vi "PC_Controller_Launcher.vi"() -> ()   [LabVIEW 2020]
doc: "PC Controller Main VI"
uses:
  TypeDefs/PosZeroOffsets.ctl
  TypeDefs/ReferenceGen.ctl
  RT Target/Controller/TypeDefs/SetRefLocEnum.ctl
  TypeDefs/PosRefOffsets.ctl
  TypeDefs/IncReference.ctl
  TypeDefs/SensorGains.ctl
  TypeDefs/AmplifierGains.ctl
  TypeDefs/CurrSenseZero.ctl
  Components_global/DynamicSignalAnalyzer/TypeDefs/ExcitationSpecs.ctl
  Components_global/DynamicSignalAnalyzer/TypeDefs/CycleSpecs.ctl
  TypeDefs/CurrSenseGains.ctl
  TypeDefs/ControllerGains_UI.ctl
  TypeDefs/ControllerGains_IndAxis.ctl
  TypeDefs/RTdisplayTimedLoop_dt.ctl
  TypeDefs/SensorHposOffset.ctl
  TypeDefs/CoordTransMultipliers.ctl
  Components_global/DynamicSignalAnalyzer/TypeDefs/DSA_TF_params.ctl
  FPGA/Components/FPGA TypeDefs/SelectDirection_Enum.ctl
  TypeDefs/BodeData.ctl
  Components/DisplayWaveform/DisplayWaveforms/DisplayWaveforms.lvclass
  C:/Program Files (x86)/National Instruments/LabVIEW 2020/vi.lib/JKI/JKI SMO/SMO/SMO.lvclass
  C:/Program Files (x86)/National Instruments/LabVIEW 2020/vi.lib/JKI/JKI SMO/SMO.UI/SMO.UI.lvclass
  Components/DisplayWaveform/DisplayWaveforms/Typedefs/Dependencies--Cluster.ctl
  RT Target/Controller/TypeDefs/STMLoopState_enum.ctl
  RT Target/Controller/TypeDefs/FuncGenParams.ctl
  FPGA/Components/FPGA TypeDefs/SelectExcitation_Enum.ctl
  Components_global/DynamicSignalAnalyzer/TypeDefs/DSAconfigCluster.ctl
  Components_global/PlannedMotionSequence/TypeDefs/PlannedMotionSequence.ctl
  Components_global/PlannedMotionSequence/TypeDefs/PlannedMotionSequence_Step.ctl
  Components_global/PlannedMotionSequence/TypeDefs/StepParams.ctl
  Components_global/PlannedMotionSequence/TypeDefs/CtrlEff Params.ctl
  Components_global/PlannedMotionSequence/TypeDefs/PosCtrl Params.ctl
  Components_global/PlannedMotionSequence/TypeDefs/HoldStateParams.ctl
  <vilib>/JKI/JKI SMO/SMO/Typedefs/SMOState --Enum.ctl
  Components_global/Queues/InterProcessQueueCtl.ctl
  TypeDefs/ConfigCluster.ctl
  TypeDefs/GraphInfoCluster.ctl
  Components_global/DynamicSignalAnalyzer/TypeDefs/BodePlot.ctl
  <vilib>/NI/STM/TCP/TCP Read Options.ctl
  <vilib>/NI/STM/TCP/Read Meta Data (TCP Ref).vi
  f38d6d6a-e512-492a-acdc-1d388213210b.vi
  78bd2656-12e6-4809-88cd-6a89556620fb.vi
  5f4b5638-6b16-4865-9ebc-64c862e354be.vi
  83d80429-4559-4d02-b91c-673944bef3a7.vi
  <vilib>/NI/STM/TCP/Get Connection Reference (TCP).vi
  <vilib>/NI/STM/TCP/Read Meta Data (TCP Clst).vi
  <vilib>/JDP Science/JSONtext/JSON text to Variant.vi
  <vilib>/JDP Science/JSONtext/Variant to JSON Text.vi
  <vilib>/NI/STM/TCP/Read Message (TCP).vi
  <vilib>/NI/STM/TCP/Write Message (TCP).vi
  <vilib>/JDP Science/JSONtext/LVClass Serializer/JSONtext LVClass Serializer.lvclass
  <vilib>/NI/STM/NI STM.lvlib
  <vilib>/JKI/JKI SMO/SMO/SMO.lvclass
  <vilib>/JKI/JKI SMO/SMO.UI/SMO.UI.lvclass
  Components_global/Queues/Queues.lvlib
  Components_global/DynamicSignalAnalyzer/DynamicSignalAnalyzer.lvlib
  <vilib>/JDP Science/JSONtext/JSONtext.lvlib
  Components_global/PlannedMotionSequence/PlannedMotionSequence.lvlib
panel:
  in  "Update Chart?":bool
  in  "Clear Chart":bool
  in  "AO Enable?":bool
  in  "Export":bool
  in  "Stop":bool
  out "Status":string
  in  "Tab Control":T1(tab)
  in  "View Raw Pos.":bool
  in  "Update Controller Gains":bool
  in  "Controller Gains":T2={"Z-direction"={"Kp"=1.0, "Ki"=0.0, "fLPF"=0.0}, "ThX-direction"={"Kp"=0.0, "Ki"=0.0, "fLPF"=0.0}, "ThY-direction"={"Kp"=0.0, "Ki"=0.0, "fLPF"=0.0}, "Bow-direction"={"Kp"=0.0, "Ki"=0.0, "fLPF"=0.0}, "B-d - direction"={"Kp"=0.0, "Ki"=0.0, "fLPF"=0.0}}
  in  "Zero Curr. Sense":bool
  in  "Set Pos. Zero":bool
  in  "Update Reference":bool
  in  "Reference Generation":T4
  in  "Run Controller?":bool
  in  "Run Plannned Motion Sequence?":bool
  in  "Sequence JSON File Path":path caption="Path"
  out "Loaded Sequence":string
  out "Bode Data":T8={"Magnitude Bode Plot"={[1.0, 1.2742749857031337, 1.6237767391887217, 2.0691380811147897, 2.636650898730358, 3.3598182862837818, 4.281332398719393, 5.455594781168519, 6.951927961775605, 8.858667904100825, 11.28837891684689, 14.38449888287663, 18.329807108324356, 23.357214690901213, 29.76351441631318, 37.926901907322495, 48.32930238571752, 61.584821106602604, 78.47599703514611, 100.0], [8.190036284839644, 6.422876871403994, 5.062364967545408, 4.022651018777153, 3.220267625701321, 2.6042578837321395, 2.1431756051838486, 1.7956979443459349, 1.5432350752401756, 1.3654027683935595, 1.2417506496398736, 1.1608055133183222, 1.1086862764056675, 1.0725909164599179, 1.0432556265245092, 1.0364066986654934, 1.0216396632894174, 1.0177430021270428, 1.0137984534990414, 1.0067815519527075]}, "Phase Bode Plot"={[1.0, 1.2742749857031337, 1.6237767391887217, 2.0691380811147897, 2.636650898730358, 3.3598182862837818, 4.281332398719393, 5.455594781168519, 6.951927961775605, 8.858667904100825, 11.28837891684689, 14.38449888287663, 18.329807108324356, 23.357214690901213, 29.76351441631318, 37.926901907322495, 48.32930238571752, 61.584821106602604, 78.47599703514611, 100.0], [-81.48463378500874, -79.51768777854348, -77.26541119865844, -74.35073441612305, -70.71358924826187, -66.32524067891468, -60.91360319984072, -54.8342286888728, -48.311197626693605, -41.59636553315517, -34.99300908851906, -29.13860750441638, -24.098834956322154, -19.566458637535703, -14.982365658719985, -13.159615969942717, -9.781179665619796, -8.18372823642157, -6.386288856595014, -4.541305979436174]}}
  in  "Meas. TF params":T9
  in  "Export DSA \ndata?":bool
  in  "Run DSA?":bool
  in  "Cycle Specs":T11={"Cycles To \nSettle (M)"=1, "Cycles To \nCalculate (N)"=2}
  in  "DSA excitation specs":T12={"Initial Freq. [Hz]"=1.0, "Final Freq. [Hz]"=100.0, "# pts. in interval"=20, "Samping Time [us]"=1000.0, "Amplitude"=0.0003, "Offset [V]"=0.0, "Freq Units (F: rad/s, T: Hz)"=TRUE}
  in  "Coord. Trans. Multipliers":T13
  in  "Sensor H-Offset  [mm]":T14={"X"=1.0, "Y"=1.0}
  in  "RT Display Reader Loop Time [us]":T15=1000 caption="Numeric"
  in  "Load\nConfig":bool
  in  "Save\nConfig":bool
  in  "Curr Sense Gain [mA/V]":T16
  in  "Curr Sense Zero [mA]":T17
  in  "Amplifier Gains [V/V]":T18={"G_SE"=1.0, "G_NE"=1.0, "G_NW"=1.0, "G_SW"=1.0, "G_CO"=1.0, "G_CI"=1.0}
  in  "Sensor Gains [um/V]":T19={"G_SE"=1.0, "G_NE"=1.0, "G_NW"=1.0, "G_SW"=1.0, "G_CI"=1.0}
  in  "Pos Zero Offsets [V]":T20
  out "# of display elements \nunpacked (row x col)":i32[](array[numeric]) caption="Numeric"
  out "FPGA Controller Loop Time [us]":dbl caption="Numeric"
  # "Planned Motion Sequence"
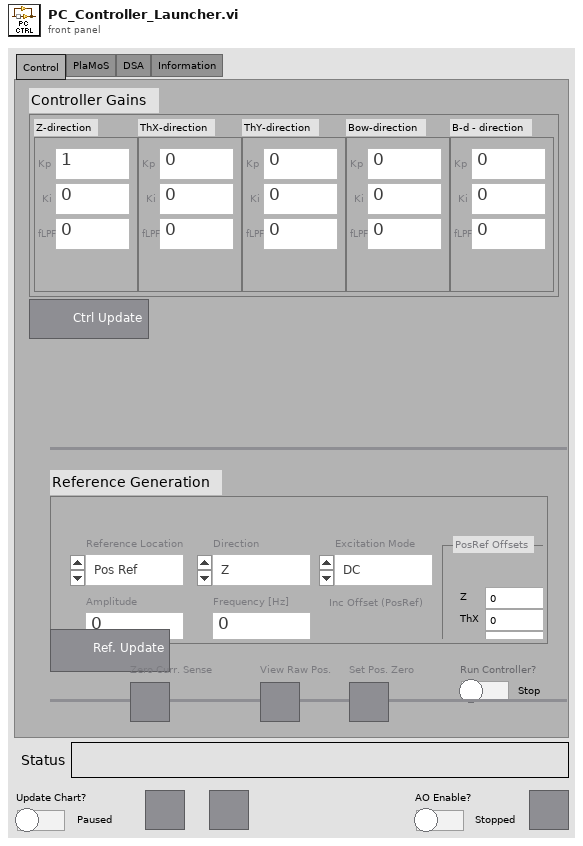
[diagram p1: front panel]
types:
  T1 = enum32{"Control", "PlaMoS", "DSA", "Information"}
  T2 = typedef "ControllerGains_UI.ctl" = cluster{"Z-direction":T3, "ThX-direction":T3, "ThY-direction":T3, "Bow-direction":T3, "B-d - direction":T3}
  T3 = typedef "ControllerGains_IndAxis.ctl" = cluster{"Kp":dbl, "Ki":dbl, "fLPF":dbl}
  T4 = typedef "ReferenceGen.ctl" = cluster{"Reference Location":T5, "Direction":enum16{"Z", "ThX", "ThY", "Bow", "B-d"}, "Excitation Mode":enum16{"DC", "Sine", "Square", "WhiteNoise"}, "Amplitude":dbl, "Frequency [Hz]":dbl, "PosRef Offsets":T6, "Inc Offset (PosRef)":T7}
  T5 = typedef "SetRefLocEnum.ctl" = enum16{"Pos Ref", "Ctrl Eff", "Elec Volt Dist"}
  T6 = typedef "PosRefOffsets.ctl" = cluster{"Z":dbl, "ThX":dbl, "ThY":dbl, "Bow":dbl, "B-d":dbl}
  T7 = typedef "IncReference.ctl" = cluster{"Step":dbl, "Arrow Up":bool, "Arrow Down":bool}
  T8 = typedef "BodeData.ctl" = cluster{"Magnitude Bode Plot":cluster{dbl[], dbl[]}, "Phase Bode Plot":cluster{dbl[], dbl[]}}
  T9 = typedef "DynamicSignalAnalyzer.lvlib/DSA_TF_params.ctl" = cluster{"Direction":T10, "Tras. Func.":enum16{"P", "RR", "C", "*_custom"}}
  T10 = typedef "SelectDirection_Enum.ctl" = enum8{"Z", "ThX", "ThY", "Bow", "B-d"}
  T11 = typedef "DynamicSignalAnalyzer.lvlib/CycleSpecs.ctl" = cluster{"Cycles To \nSettle (M)":i16, "Cycles To \nCalculate (N)":i16}
  T12 = typedef "DynamicSignalAnalyzer.lvlib/ExcitationSpecs.ctl" = cluster{"Initial Freq. [Hz]":dbl, "Final Freq. [Hz]":dbl, "# pts. in interval":i16, "Samping Time [us]":dbl, "Amplitude":dbl, "Offset [V]":dbl, "Freq Units (F: rad/s, T: Hz)":bool}
  T13 = typedef "CoordTransMultipliers.ctl" = cluster{"Z":dbl, "Th":dbl}
  T14 = typedef "SensorHposOffset.ctl" = cluster{"X":dbl, "Y":dbl}
  T15 = typedef "RTdisplayTimedLoop_dt.ctl" = i64
  T16 = typedef "CurrSenseGains.ctl" = cluster{"G_CS":dbl}
  T17 = typedef "CurrSenseZero.ctl" = cluster{"I_SE":dbl, "I_NE":dbl, "I_NW":dbl, "I_SW":dbl, "I_CO":dbl, "I_CI":dbl}
  T18 = typedef "AmplifierGains.ctl" = cluster{"G_SE":dbl, "G_NE":dbl, "G_NW":dbl, "G_SW":dbl, "G_CO":dbl, "G_CI":dbl}
  T19 = typedef "SensorGains.ctl" = cluster{"G_SE":dbl, "G_NE":dbl, "G_NW":dbl, "G_SW":dbl, "G_CI":dbl}
  T20 = typedef "PosZeroOffsets.ctl" = cluster{"V_SE":dbl, "V_NE":dbl, "V_NW":dbl, "V_SW":dbl, "V_CI":dbl}
  T21 = typedef "STMLoopState_enum.ctl" = enum16{"Initialize", "Warm-up", "Run", "ShutDown"}
  T22 = typedef "DisplayWaveform.lvlib/DisplayWaveforms.lvclass/Dependencies--Cluster.ctl" = cluster{"New Value":refnum<user-event>}
  T23 = typedef "SMO.lvclass/Public Events.ctl" = cluster{"Error":refnum<user-event>, "State":refnum<user-event>, "Reserve State":refnum<user-event>}
  T24 = typedef "SMO.UI.lvclass/PublicEvents--Cluster.ctl" = cluster{"UI Hidden":refnum<user-event>, "UI State":refnum<user-event>}
  T25 = typedef "DisplayWaveform.lvlib/DisplayWaveforms.lvclass/PublicEvents--Cluster.ctl" = cluster{"Chart Cleared":refnum<user-event>, "Chart Exported":refnum<user-event>, "ChartParams Set":refnum<user-event>}
  T26 = typedef "NI STM.lvlib/TCP Connection Info.ctl" = cluster{"connection ID":refnum<k5>, "meta data":T27[]}
  T27 = typedef "NI STM.lvlib/MetaDataElement.ctl" = string
  T28 = typedef "Queues.lvlib/Queue Refs.ctl" = cluster{"InterProcessQueue":refnum<queue>}
  T29 = typedef "SMO.lvclass/SMOState --Enum.ctl" = enum16{"unknown", "Created", "Started", "Stopped"}
  T30 = enum32{"Invalid", "Standard", "Closed", "Hidden", "Minimized", "Maximized"}
  T31 = enum32{"invalid app kind", "Development System", "Run Time System", "Student Edition", "Embedded LabVIEW", "Evaluation", "Custom"}
  T32 = typedef "Queues.lvlib/InterProcessQueueCtl.ctl" = cluster{"Command":string, "Data":variant}
  T33 = typedef "FuncGenParams.ctl" = cluster{"Reference Location":T5, "Direction":T10, "Excitation mode":T34, "Amplitude":dbl, "Frequency (periods/tick)":dbl, "PosRef_Offset":dbl[]}
  T34 = typedef "SelectExcitation_Enum.ctl" = enum8{"DC", "Sine", "Square", "WhiteNoise"}
  T35 = enum8{"Enabled", "Disabled", "Disabled and Grayed Out"}
  T36 = typedef "DynamicSignalAnalyzer.lvlib/DSAconfigCluster.ctl" = cluster{"DSA excitation specs":T12, "Cycle Specs":T11, "Meas. TF params":T9}
  T37 = typedef "ConfigCluster.ctl" = cluster{"Controller Gains":T2, "Reference Generation":T4, "RT Display Reader Loop Time [us]":i64, "Sensor Gains [um/V]":T19, "Amplifier Gains [V/V]":T18, "Curr Sense Gain [mA/V]":T16, "Sensor Offset  [mm]":T14, "Coord. Trans. Multipliers":T13, "DSA Config Cluster":T36, "Pos Zero Offsets [V]":T20}
  T38 = enum16{"open", "replace", "create", "open or create", "replace or create", "replace or create with confirmation"}
  T39 = typedef "GraphInfoCluster.ctl" = cluster{"RT Display Reader Loop Time [us]":T15, "Sensor Gains [um/V]":T19, "Sensor H-Offset  [mm]":T14, "Amplifier Gains [V/V]":T18, "Curr Sense Gain [mA/V]":T16}
  T40 = typedef "DynamicSignalAnalyzer.lvlib/BodePlot.ctl" = cluster{"Frequency [Hz]":dbl[], "Magnitude [abs]":dbl[], "Phase [deg]":dbl[]}
  T41 = typedef "PlannedMotionSequence.lvlib/PlannedMotionSequence.ctl" = T42[]
  T42 = typedef "PlannedMotionSequence.lvlib/PlannedMotionSequence_Step.ctl" = cluster{"_Comment":string, "StepParams":T43, "Controller Gains":T2}
  T43 = typedef "PlannedMotionSequence.lvlib/StepParams.ctl" = cluster{"Ctrl State":enum16{"PosCtrl", "CtrlEff", "HoldState"}, "CtrlEff Params":T44, "PosCtrl Params":T45, "HoldState Params":T46}
  T44 = typedef "PlannedMotionSequence.lvlib/CtrlEff Params.ctl" = cluster{"Time [s]":dbl, "U_z":dbl}
  T45 = typedef "PlannedMotionSequence.lvlib/PosCtrl Params.ctl" = cluster{"Velocity [um/s]":dbl, "Starting Z-position [um]":dbl, "Ending Z-position [um]":dbl, "Bow Reference [um]":dbl}
  T46 = typedef "PlannedMotionSequence.lvlib/HoldStateParams.ctl" = cluster{"Time [s]":dbl}
  T47 = cluster{"Core":cluster{"Current VI Reference":refnum<vi>, "Close Panel on Exit?":bool}, "UI switch state":bool, "Export Folder Path":path}
  T48 = cluster{"PosRef Offsets[0]":dbl, "PosRef Offsets[1]":dbl, "PosRef Offsets[2]":dbl, "PosRef Offsets[3]":dbl, "PosRef Offsets[4]":dbl}
  T49 = cluster{"Current VI Reference":refnum<vi>, "Close Panel on Exit?":bool}
  T50 = typedef "ChartParamsCluster.ctl" = cluster{"Chart ScaleMultipliers":cluster{"WF Xscale Multiplier":dbl, "WF Yscale Multiplier":dbl[]}, "Coord Transform Multipliers":cluster{"Z-Multiplier":dbl, "Th-Multiplier":dbl}}
  T51 = typedef "imagedata.ctl" = cluster{"image type":i32, "image depth":i32, "image":u8[], "mask":u8[], "colors":u32[], "Rectangle":cluster{"left":i16, "top":i16, "right":i16, "bottom":i16}}
  T52 = typedef "NI STM.lvlib/TCP Read Options.ctl" = cluster{"ignore timeout error":bool, "timeout ms (1000)":i32}
  T53 = cluster{"V_SE":dbl, "V_NE":dbl, "V_NW":dbl, "V_SW":dbl, "V_CI":dbl}
  T54 = cluster{"I_SE":dbl, "I_NE":dbl, "I_NW":dbl, "I_SW":dbl, "I_CO":dbl, "I_CI":dbl}
  T55 = cluster{"Frequency [Hz]":dbl[], "Magnitude [abs]":dbl[]}
  T56 = cluster{"Frequency [Hz]":dbl[], "Phase [deg]":dbl[]}
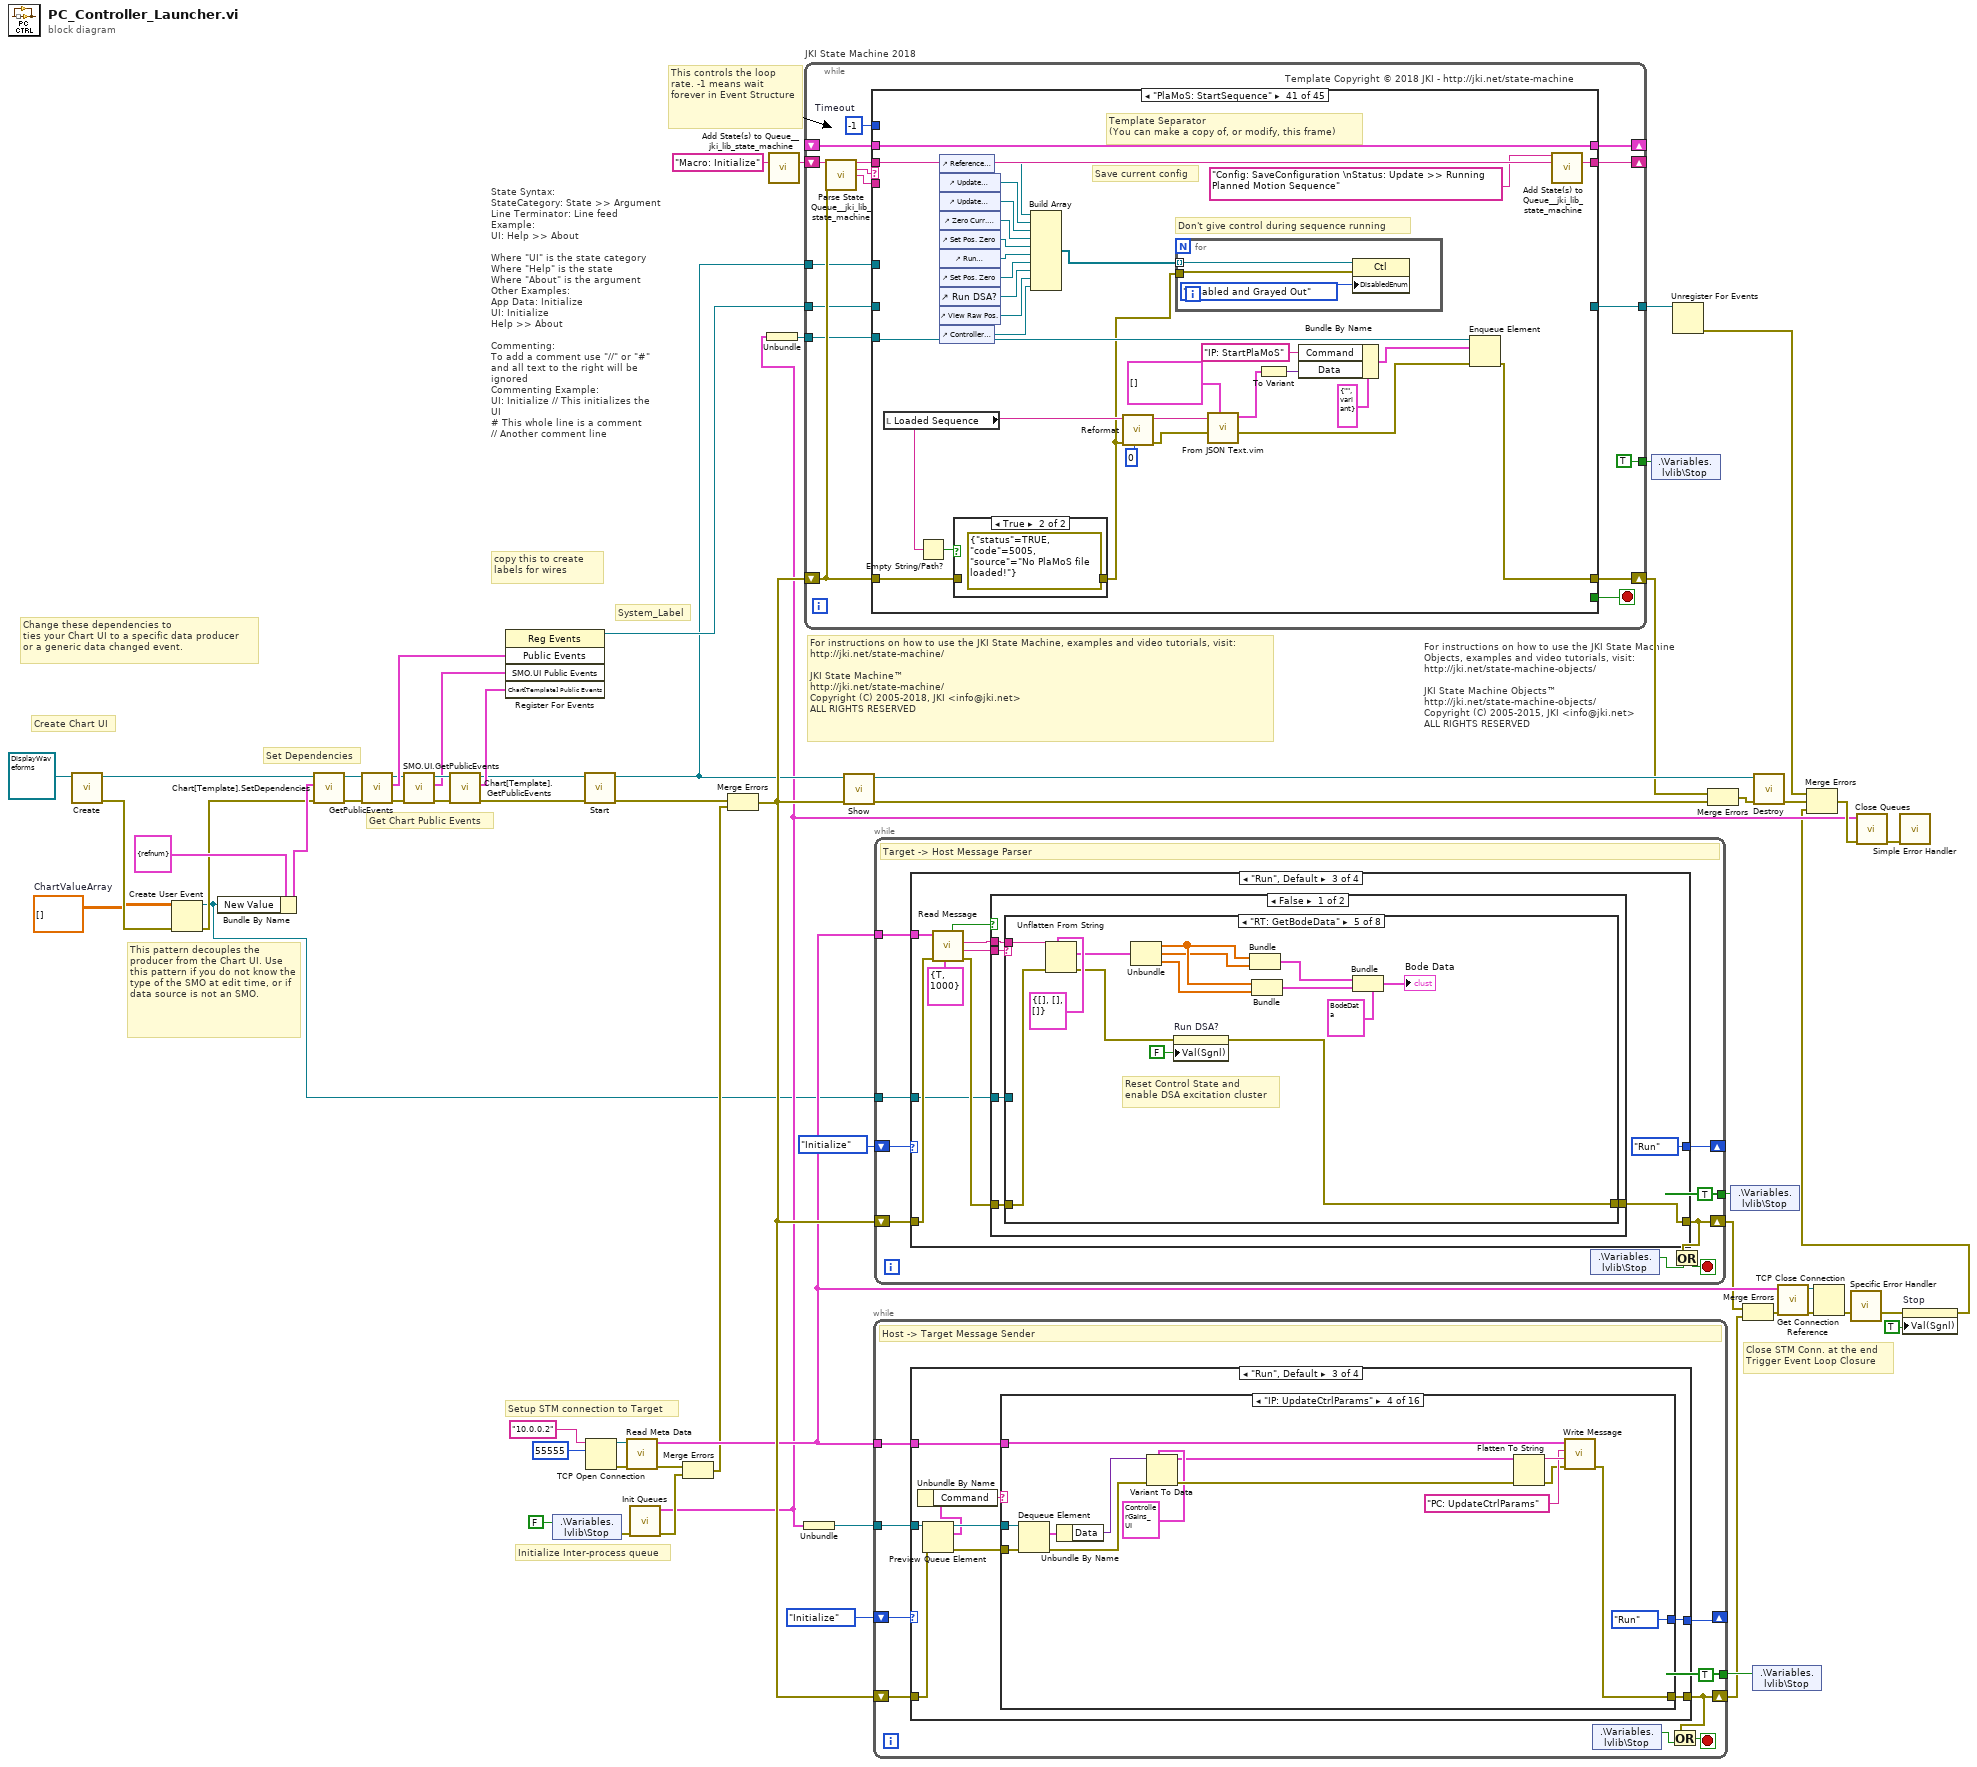
[diagram p0: block diagram]
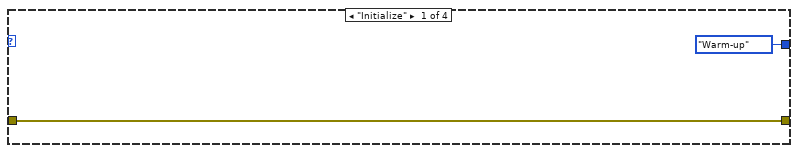
[diagram p2: hidden frame]
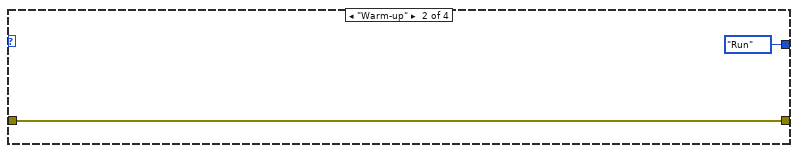
[diagram p3: hidden frame]
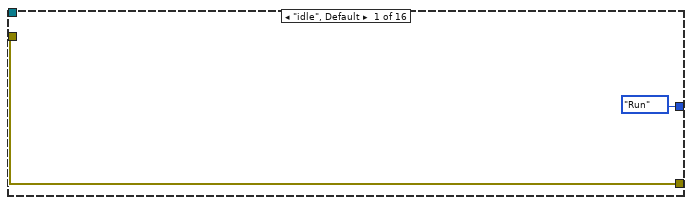
[diagram p4: hidden frame]
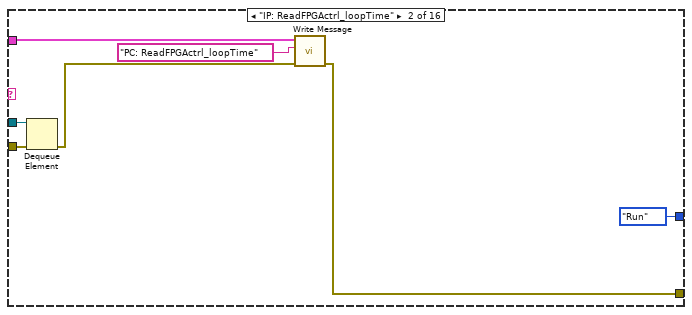
[diagram p5: hidden frame]
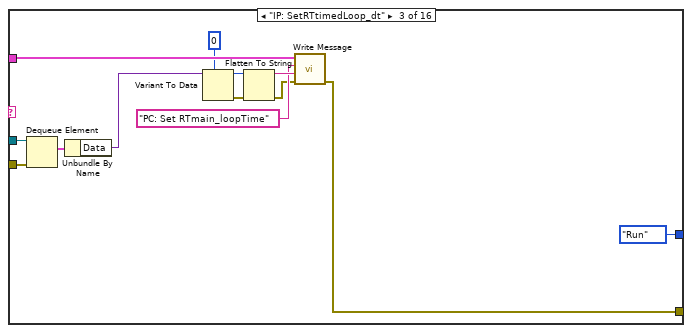
[diagram p6: hidden frame]
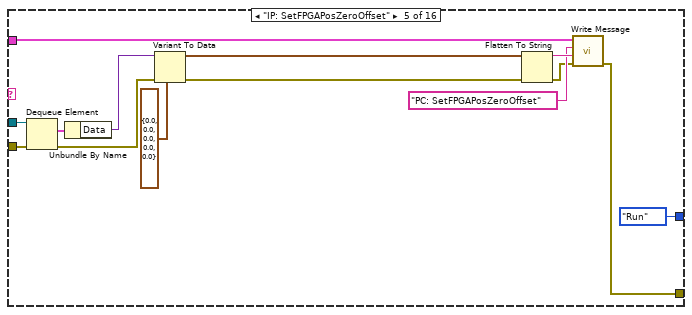
[diagram p7: hidden frame]
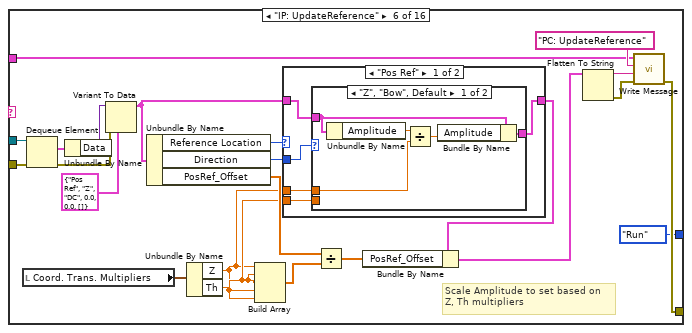
[diagram p8: hidden frame]
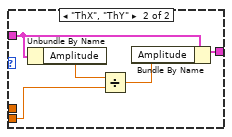
[diagram p9: hidden frame]
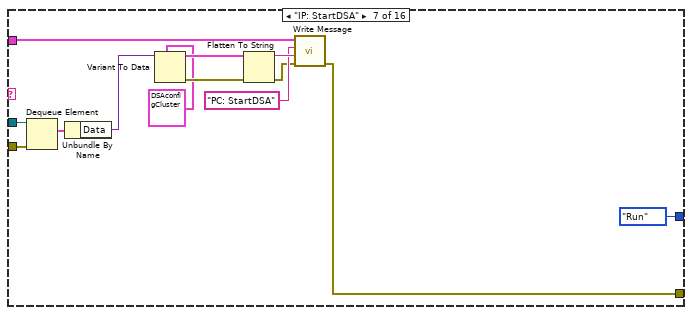
[diagram p11: hidden frame]
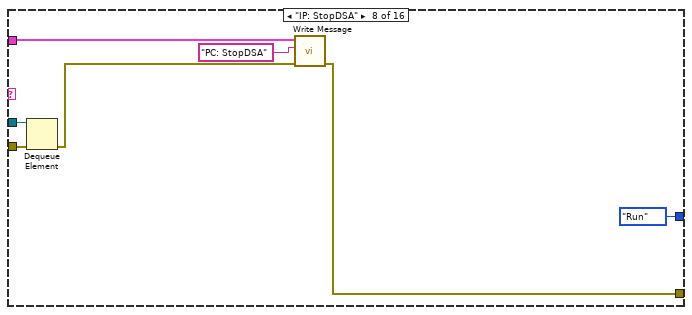
[diagram p12: hidden frame]
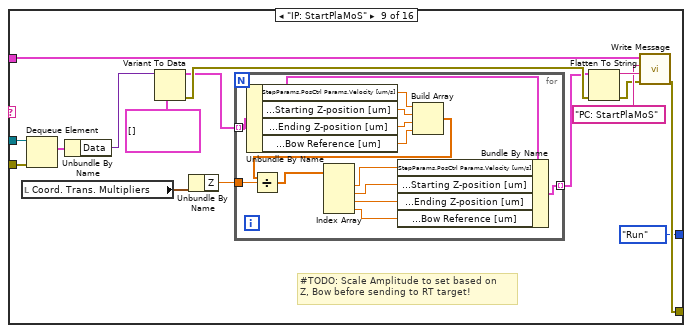
[diagram p13: hidden frame]
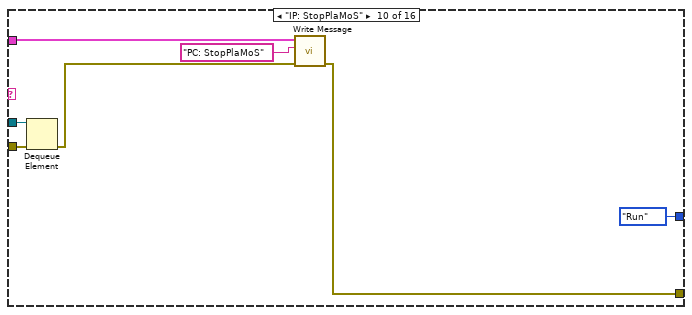
[diagram p14: hidden frame]
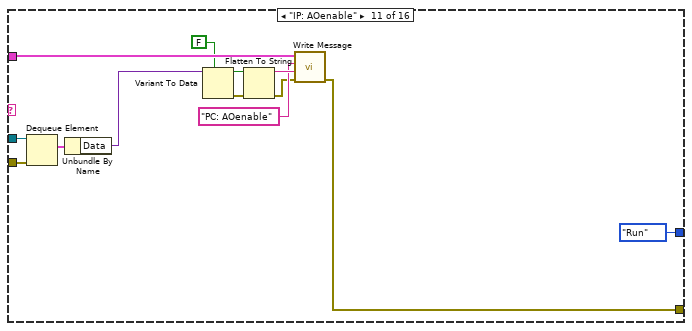
[diagram p15: hidden frame]
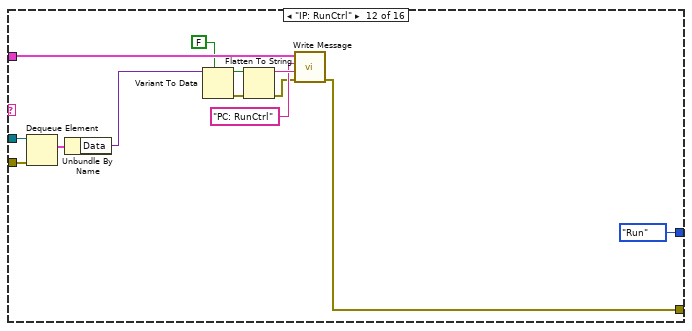
[diagram p16: hidden frame]
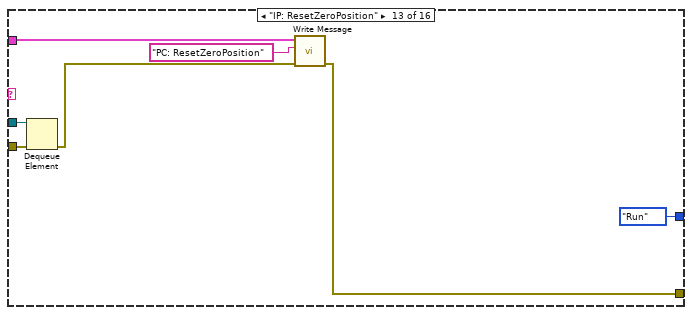
[diagram p17: hidden frame]
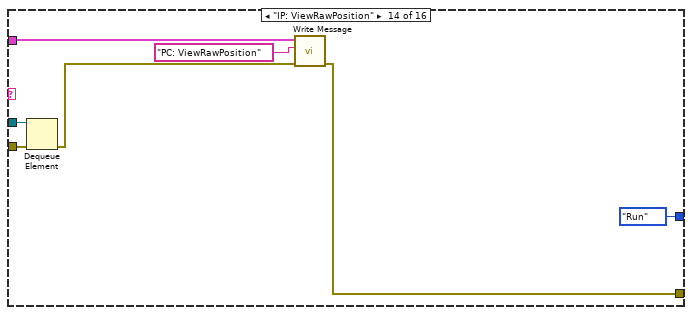
[diagram p18: hidden frame]
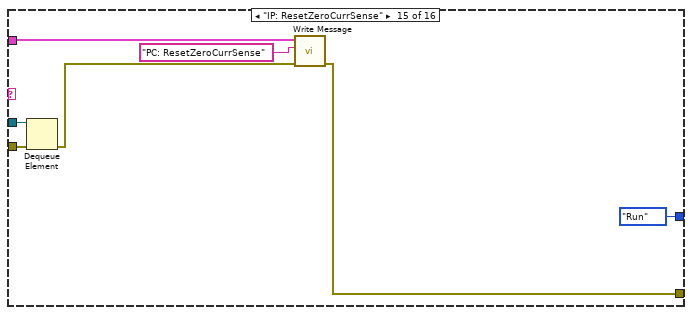
[diagram p19: hidden frame]
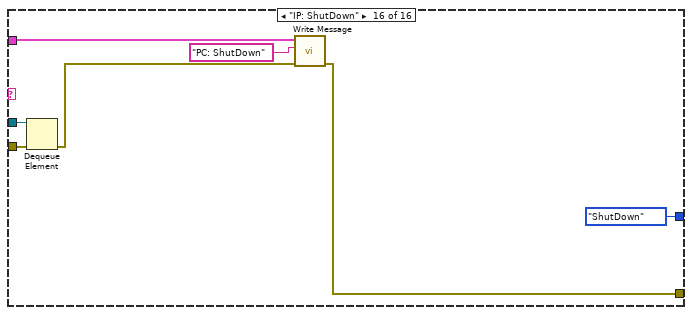
[diagram p20: hidden frame]
diagram:
  w6 = dbl[][] []  # ChartValueArray
  # "Close STM Conn. at the end\nTrigger Event Loop Closure"
  # "Setup STM connection to Target"
  # "Initialize Inter-process queue"
  # "This pattern decouples the producer from the Chart UI. Use this pattern if you do not know the type of the SMO at edit time, or if data source is not an SMO."
  # "For instructions on how to use the JKI State Machine, examples and video tutorials, visit:\nhttp://jki.net/state-machine/\n\nJKI State Machine™\nhttp://jki.net/state-machine/\nCopyright (C) 2005-2018, JKI <info@jki.net>\nALL RIGHTS RESERVED"
  # "State Syntax:\nStateCategory: State >> Argument\nLine Terminator: Line feed\nExample:\nUI: Help >> About\n\nWhere \"UI\" is the state category\nWhere \"Help\" is the state\nWhere \"About\" is the argument\nOther Examples:\nApp Data: Initialize\nUI: Initialize\nHelp >> About\n\nCommenting:\nTo add a comment use \"//\" or \"#\" and all text to the right will be ignored\nCommenting Example:\nUI: Initialize // This initializes the UI\n# This whole line is a comment\n// Another comment line"
  # "copy this to create labels for wires"
  # "This controls the loop rate. -1 means wait forever in Event Structure"
  # "System_Label"
  # "Set Dependencies"
  # "Create Chart UI"
  # "Change these dependencies to\nties your Chart UI to a specific data producer\nor a generic data changed event."
  # "For instructions on how to use the JKI State Machine Objects, examples and video tutorials, visit:\nhttp://jki.net/state-machine-objects/\n\nJKI State Machine Objects™\nhttp://jki.net/state-machine-objects/\nCopyright (C) 2005-2015, JKI <info@jki.net>\nALL RIGHTS RESERVED"
  # "Get Chart Public Events"
  n1 = call <vilib>:"Create.vi"("SMO"=refnum<class "DisplayWaveforms.lvclass"> refnum ("Chart[Template]")) -> ("error out"=w8:errorcluster, "SMO out"=w53:refnum<class "DisplayWaveforms.lvclass">)  [unwired: 8 in, 1 out]
  n2 = Create User Event(user event datatype=w6, error in=w8) -> (user event=w5:refnum<user-event>, error out=w7:errorcluster)
  n3 = Bundle By Name(cluster=T22 {"New Value"=refnum} ("Dependencies"), "New Value"=w5) -> (w51:T22)
  n4 = call "Chart[Template].SetDependencies.vi"("error in (no error)"=w7, "Dependencies"=w51, "DisplayWaveforms"=w53) -> ("error out"=w39:errorcluster, "DisplayWaveforms out"=w50:refnum<class "DisplayWaveforms.lvclass">)  [unwired: 7 in]
  n5 = call <vilib>:"GetPublicEvents.vi"("error in (no error)"=w39, "SMO"=w50) -> ("error out"=w45:errorcluster, "Public Events"=w49:T23, "SMO out"=w47:refnum<class "DisplayWaveforms.lvclass">)  [unwired: 7 in]
  n6 = call <vilib>:"SMO.UI.GetPublicEvents.vi"("error in (no error)"=w45, "SMO.UI"=w47) -> ("error out"=w44:errorcluster, "SMO.UI Public Events"=w43:T24, "SMO.UI out"=w46:refnum<class "DisplayWaveforms.lvclass">)  [unwired: 7 in]
  n7 = call "Chart[Template].GetPublicEvents.vi"("error in (no error)"=w44, "DisplayWaveforms"=w46) -> ("error out"=w40:errorcluster, "Chart[Template] Public Events"=w48:T25, "DisplayWaveforms out"=w41:refnum<class "DisplayWaveforms.lvclass">)  [unwired: 7 in]
  n8 = register-events(w49, w43, w48) -> (reference out=w42:refnum<event-registration>)  [unwired: 2 in, 1 out]
  n9 = shared-variable ".\\Variables.lvlib\\Stop"(FALSE ("Stop")) -> (error out=w30:errorcluster)  [unwired: 1 in]
  n10 = call <vilib>:"Start.vi"("error in (no error)"=w40, "SMO"=w41) -> ("error out"=w25:errorcluster, "SMO out"=w23:refnum<class "DisplayWaveforms.lvclass">)  [unwired: 8 in]
  n11 = TCP Open Connection(address="10.0.0.2" ("Target IP Address"), remote port or service name=u16 55555 ("remote port")) -> (connection ID=w61:refnum<k5>, error out=w60:errorcluster)  [unwired: 1 in, 2 out]
  n12 = call-poly <vilib>:"Read Meta Data.vi"("error in"=w60, "connection ID"=w61) -> ("error out"=w13:errorcluster, "connection info out"=w19:T26)  [unwired: 1 in, 7 out]
  n13 = call "Init Queues.vi"("error in (no error)"=w30) -> ("error out"=w12:errorcluster, "Queue Refs"=w9:T28)  [unwired: 9 in]
  n14 = Merge Errors(w13, w12) -> (w11:errorcluster)
  n15 = Merge Errors(w25, w11) -> (w24:errorcluster)
  n16 = Unbundle(w9) -> ("InterProcessQueue"=w10:refnum<queue>)
  n17 = call <vilib>:"Add State(s) to Queue__jki_lib_state_machine.vi"("State(s) in (\"\")"="Macro: Initialize") -> ("States Out"=w37:string)  [unwired: 14 in]
  n18 = Unbundle(w9) -> ("InterProcessQueue"=w26:refnum<queue>)
  n19 = while "JKI State Machine 2018" {
    shift-right: [w64] -> _
    shift-left: _ -> [w70]
    shift-right: [w72] -> _
    shift-left: w37 -> [w74]
    tunnel: w42 -> [w67]
    tunnel: w23 -> [w66]
    tunnel: [w65] -> w35
    tunnel: [TRUE ("Stop")] -> w33
    shift-right: [w73] -> w4
    shift-left: w24 -> [w68]
    tunnel: w10 -> [w62]
    stop <- w71 stop-if-true
    w69 = -1  # Timeout
    # "Template Copyright © 2018 JKI - http://jki.net/state-machine"
    n20 = call <vilib>:"Parse State Queue__jki_lib_state_machine.vi"("State Queue"=w74, "Error In (no error)"=w68) -> ("Remaining States"=w76:string, "Current State"=w77:string, "Arguments"=w75:string)  [unwired: 11 in]
    n21 = case shown="\"PlaMoS: StartSequence\"" w77 {
      selector: w77 -> [_ _ w279 _ _ _ _ _ _ _ _ _ _ _ _ _ _ _ _ _ _ _ _ _ _ _ _ _ _ _ _ _ _ _ _ _ _ _ _ _ _ _ _ _ _]
      tunnel: w76 -> [w88 w278 w283 w302 w304 w316 w320 w327 w333 w337 w345 w354 w365 w434 w443 w455 w469 w483 w493 w503 w513 w525 w537 w560 w577 w599 w604 w621 w625 w661 w696 w718 w725 w734 w738 w743 w765 w769 w787 w811 w842 w869 w877 w881 w885]
      tunnel: w75 -> [_ _ _ _ _ _ _ _ _ _ _ w349 w359 _ _ _ _ _ _ _ _ _ _ _ _ _ _ _ _ _ w667 _ _ w726 _ _ _ _ _ _ _ _ _ _ _]
      tunnel: w70 -> [w86 w275 w281 w295 w308 w314 w317 _ w328 w334 w343 w352 w361 w431 w437 w453 w460 w471 w491 w501 w511 w523 w535 w558 w571 w596 w601 w619 w622 w659 w666 w721 w722 w731 w735 w740 w762 w766 w785 w809 w840 w867 w874 w878 w882]
      tunnel: [w85 w276 w285 w299 errorcluster {"status"=FALSE, "code"=0, "source"=""} ("error out") w313 w318 w324 w329 w335 w338 w350 w362 w432 w435 w445 w456 w473 w487 w497 w507 w516 w528 w539 w572 w597 w602 w606 w623 w644 w681 w713 w723 w732 w736 w741 w745 w767 w773 w804 w828 w860 w875 w879 w883] -> w73
      tunnel: w68 -> [w84 w276 w284 w299 w307 w313 w318 w324 w330 w335 w340 w351 w363 w432 w436 w446 w457 w474 w486 w496 w506 w517 w529 w540 w573 w597 w602 w608 w623 w654 w682 w714 w723 w732 w736 w741 w761 w767 w775 w804 w824 w861 w875 w879 w883]
      tunnel: [w87 w277 w282 w301 w310 w315 w319 w326 w332 w336 w344 w353 w364 w433 w442 w454 w468 w482 w492 w502 w512 w524 w536 w559 w576 w598 w603 w620 w624 w660 w695 w719 w724 w733 w737 w742 w764 w768 w786 w810 w841 w868 w876 w880 w884] -> w72
      tunnel: [_ _ _ _ _ TRUE _ _ _ _ _ _ _ _ _ _ _ _ _ _ _ _ _ _ _ _ _ _ _ _ _ _ _ _ _ _ _ _ _ _ _ _ _ _ _] -> w71
      tunnel: [w83 w275 w281 w300 w308 w314 w317 w325 w328 w334 w343 w352 w361 w431 w437 w453 w460 w471 w491 w501 w511 w523 w535 w558 w571 w596 w601 w619 w622 w659 w666 w721 w722 w731 w735 w740 w762 w766 w785 w809 w840 w867 w874 w878 w882] -> w64
      tunnel: w69 -> [w82 _ _ _ _ _ _ _ _ _ _ _ _ _ _ _ _ _ _ _ _ _ _ _ _ _ _ _ _ _ _ _ _ _ _ _ _ _ _ _ _ _ _ _ _]
      tunnel: w67 -> [w81 _ _ _ _ w311 _ _ _ _ _ _ _ _ _ _ _ _ _ _ _ _ _ _ _ _ _ _ _ _ _ _ _ _ _ _ _ _ _ _ _ _ _ _ _]
      tunnel: w66 -> [w80 _ _ _ _ _ _ _ _ _ _ _ _ _ _ _ _ _ _ _ _ _ _ _ _ _ _ _ _ _ _ w717 _ _ _ _ _ _ _ _ _ _ _ _ _]
      tunnel: [w79 _ _ _ _ w311 _ _ _ _ _ _ _ _ _ _ _ _ _ _ _ _ _ _ _ _ _ _ _ _ _ _ _ _ _ _ _ _ _ _ _ _ _ _ _] -> w65
      tunnel: w62 -> [w78 _ _ _ _ _ _ _ _ _ _ _ _ _ w438 w447 w461 w475 w485 w495 w505 w518 w530 w542 w574 _ _ w605 _ _ _ _ _ _ _ _ _ _ _ _ w834 w864 _ _ _]
      frame "", "Event Structure", "Idle" {
        # "executes when the state queue is empty"
        n22 = event shown="[16] \"Load Config\": Value Change" {
          selector: w81 -> [_ _ _ _ _ _ _ _ _ _ _ _ _ _ _ _ _ _ _ _ _ _ _]
          dyn-events: [_ _ _ _ _ _ _ _ _ _ _ _ _ _ _ _ _ _ _ _ _ _ _] -> w79
          timeout: w82 -> [_ _ _ _ _ _ _ _ _ _ _ _ _ _ _ _ _ _ _ _ _ _ _]
          tunnel: w88 -> [w92 w98 w105 w109 w114 w119 w124 w129 w147 w165 w173 w179 w194 w204 w211 w215 w220 w228 w237 w249 w259 w263 w270]
          tunnel: [w91 w99 w106 w110 w115 w120 w125 w130 w148 w166 w172 w178 w193 w203 w212 w216 w221 w229 w236 w248 w258 w262 w270] -> w87
          tunnel: w86 -> [w89 w97 w104 w111 w116 w121 w126 w131 w149 w167 w174 w181 w189 w201 w210 w217 w222 w227 w233 w247 w257 w264 w271]
          tunnel: [w90 w93 w101 w107 w112 w117 w123 w128 w146 w164 w175 w182 w196 w202 w207 w213 w218 w224 w230 w239 w250 w265 w272] -> w85
          tunnel: w84 -> [w90 w93 w101 w107 w112 w117 w123 w128 w146 w164 w176 w183 w190 w202 w207 w213 w218 w224 w234 w242 w251 w265 w273]
          tunnel: [w89 w95 w103 w111 w116 w121 w126 w131 w149 w167 w174 w181 w187 w201 w209 w217 w222 w226 w231 w247 w257 w264 w271] -> w83
          tunnel: w80 -> [_ _ _ _ _ _ _ _ _ _ w177 w184 w192 _ _ _ _ _ w235 w243 w252 _ w274]
          tunnel: w78 -> [_ _ _ _ _ _ _ _ _ _ _ _ _ _ _ _ _ _ _ _ _ _ _]
          event Timeout {
            # "README FIRST\nThis VI template should be used by dragging & dropping it from the Functions palette onto the Block Diagram of a new, blank VI, which will place it's contents into the blank VI.\n\nDo not edit the VI found in the palette.  Only edit the state machine after it is placed into your blank VI.\n\nFor instructions on how to use the JKI State Machine, examples and video tutorials, visit:\nhttp://jki.net/state-machine/\n\nDELETE THIS NOTE AFTER READING"
            # "Timeout Frame\n(this will only execute if the Event Structure timeout is >= 0)"
            n23 = event-data() -> ()  [unwired: 1 in, 1 out]
            n24 = call <vilib>:"Add State(s) to Queue__jki_lib_state_machine.vi"("State(s) in (\"\")"=w92) -> ("States Out"=w91:string)  [unwired: 14 in]
          }
          event "AO Enable?": Value Change {
            n25 = event-data() -> ("NewVal"=w96:bool)  [unwired: 1 in, 5 out]
            n26 = Bundle By Name(cluster=w97, "UI switch state"=w96) -> (w95:T47)
            n27 = call <vilib>:"Add State(s) to Queue__jki_lib_state_machine.vi"("State(s) in Front (\"\")"="IP: AOenable" ("State(s) in Front (\"\")"), "State(s) in (\"\")"=w98) -> ("States Out"=w99:string)  [unwired: 13 in]
          }
          event "Run Controller?": Value Change {
            n28 = event-data() -> ("NewVal"=w102:bool)  [unwired: 1 in, 5 out]
            n29 = Bundle By Name(cluster=w104, "UI switch state"=w102) -> (w103:T47)
            n30 = call <vilib>:"Add State(s) to Queue__jki_lib_state_machine.vi"("State(s) in Front (\"\")"="IP: RunController" ("State(s) in Front (\"\")"), "State(s) in (\"\")"=w105) -> ("States Out"=w106:string)  [unwired: 13 in]
          }
          event "Set Pos. Zero": Value Change {
            n31 = event-data() -> ()  [unwired: 1 in, 6 out]
            n32 = call <vilib>:"Add State(s) to Queue__jki_lib_state_machine.vi"("State(s) in Front (\"\")"="IP: ResetZeroPosition", "State(s) in (\"\")"=w109) -> ("States Out"=w110:string)  [unwired: 13 in]
          }
          event "View Raw Pos.": Value Change {
            n33 = event-data() -> ()  [unwired: 1 in, 6 out]
            n34 = call <vilib>:"Add State(s) to Queue__jki_lib_state_machine.vi"("State(s) in Front (\"\")"="IP: ViewRawPosition", "State(s) in (\"\")"=w114) -> ("States Out"=w115:string)  [unwired: 13 in]
          }
          event "Zero Curr. Sense": Value Change {
            n35 = event-data() -> ()  [unwired: 1 in, 6 out]
            n36 = call <vilib>:"Add State(s) to Queue__jki_lib_state_machine.vi"("State(s) in Front (\"\")"="IP: ResetZeroCurrSense", "State(s) in (\"\")"=w119) -> ("States Out"=w120:string)  [unwired: 13 in]
          }
          event "Update Controller Gains": Value Change {
            n37 = event-data() -> ()  [unwired: 1 in, 6 out]
            n38 = call <vilib>:"Add State(s) to Queue__jki_lib_state_machine.vi"("State(s) in Front (\"\")"="IP: UpdateCtrlGains", "State(s) in (\"\")"=w124) -> ("States Out"=w125:string)  [unwired: 13 in]
          }
          event "Update Reference": Value Change {
            n39 = event-data() -> ()  [unwired: 1 in, 6 out]
            n40 = call <vilib>:"Add State(s) to Queue__jki_lib_state_machine.vi"("State(s) in Front (\"\")"="IP: UpdateReference" ("State(s) in Front (\"\")"), "State(s) in (\"\")"=w129) -> ("States Out"=w130:string)  [unwired: 13 in]
          }
          event Value Change {
            n41 = event-data() -> ()  [unwired: 1 in, 6 out]
            n42 = local read "Reference Generation"() -> (w140:T4)
            n43 = Unbundle By Name(w140) -> ("PosRef Offsets"=w144:T6, "Direction"=w142:enum16{"Z", "ThX", "ThY", "Bow", "B-d"}, "Inc Offset (PosRef).Step"=w135:dbl)
            n44 = property on="Reference Generation" class="Clust (strict)"() -> ("Value"=w134:T4)  [unwired: 2 in, 2 out]
            n45 = Bundle By Name(cluster=w134, "Inc Offset (PosRef).Arrow Up"=FALSE ("Inc. Offset.Arrow Down")) -> (w133:T4)
            n46 = Cluster To Array(cluster=w144) -> (array=w143:dbl[])
            n47 = Index Array(array=w143, index=w142) -> (element=w136:dbl)
            n48 = Add(x=w136, y=w135) -> (x+y=w141:dbl)
            n49 = Replace Array Subset(array=w143, new element=w141, index=w142) -> (w139:dbl[])
            n50 = Array To Cluster(array=w139) -> (cluster=w138:T48)
            n51 = Bundle By Name(cluster=w140, "PosRef Offsets"=w138) -> (w137:T4)
            n52 = property on="Reference Generation" class="Clust (strict)"("Value"=w133) -> ()  [unwired: 2 in, 2 out]
            n53 = local write "Reference Generation"(w137) -> ()
            n54 = call <vilib>:"Add State(s) to Queue__jki_lib_state_machine.vi"("State(s) in Front (\"\")"="IP: UpdateReference" ("State(s) in Front (\"\")"), "State(s) in (\"\")"=w147) -> ("States Out"=w148:string)  [unwired: 13 in]
          }
          event Value Change {
            n55 = event-data() -> ()  [unwired: 1 in, 6 out]
            n56 = local read "Reference Generation"() -> (w158:T4)
            n57 = Unbundle By Name(w158) -> ("PosRef Offsets"=w162:T6, "Direction"=w160:enum16{"Z", "ThX", "ThY", "Bow", "B-d"}, "Inc Offset (PosRef).Step"=w153:dbl)
            n58 = property on="Reference Generation" class="Clust (strict)"() -> ("Value"=w152:T4)  [unwired: 2 in, 2 out]
            n59 = Cluster To Array(cluster=w162) -> (array=w161:dbl[])
            n60 = Bundle By Name(cluster=w152, "Inc Offset (PosRef).Arrow Down"=FALSE ("Inc. Offset.Arrow Down")) -> (w151:T4)
            n61 = Index Array(array=w161, index=w160) -> (element=w154:dbl)
            n62 = Subtract(x=w154, y=w153) -> (x-y=w159:dbl)
            n63 = Replace Array Subset(array=w161, new element=w159, index=w160) -> (w157:dbl[])
            n64 = Array To Cluster(array=w157) -> (cluster=w156:T48)
            n65 = Bundle By Name(cluster=w158, "PosRef Offsets"=w156) -> (w155:T4)
            n66 = property on="Reference Generation" class="Clust (strict)"("Value"=w151) -> ()  [unwired: 2 in, 2 out]
            n67 = local write "Reference Generation"(w155) -> ()
            n68 = call <vilib>:"Add State(s) to Queue__jki_lib_state_machine.vi"("State(s) in Front (\"\")"="IP: UpdateReference" ("State(s) in Front (\"\")"), "State(s) in (\"\")"=w165) -> ("States Out"=w166:string)  [unwired: 13 in]
          }
          event "Update Chart?": Value Change {
            n69 = event-data() -> ("NewVal"=w168:bool)  [unwired: 1 in, 5 out]
            n70 = call "UpdateChart.vi"("error in (no error)"=w176, "Update Chart?"=w168, "DisplayWaveforms"=w177) -> ("error out"=w175:errorcluster)  [unwired: 7 in, 1 out]
            n71 = Select(t="Status: Update >> Charts Update Running" ("State(s) in Front (\"\")"), s=w168, f="Status: Update >> Charts Update Paused" ("State(s) in Front (\"\")")) -> (s? t:f=w169:string)
            n72 = call <vilib>:"Add State(s) to Queue__jki_lib_state_machine.vi"("State(s) in Front (\"\")"=w169, "State(s) in (\"\")"=w173) -> ("States Out"=w172:string)  [unwired: 13 in]
          }
          event "Clear Chart": Value Change {
            # "Send Data to UI"
            n73 = event-data() -> ()  [unwired: 1 in, 6 out]
            n74 = call "Clear Chart.vi"("error in (no error)"=w183, "DisplayWaveforms"=w184) -> ("error out"=w182:errorcluster)  [unwired: 8 in, 1 out]
            n75 = call <vilib>:"Add State(s) to Queue__jki_lib_state_machine.vi"("State(s) in Front (\"\")"="Status: Update >> Charts cleared" ("State(s) in Front (\"\")"), "State(s) in (\"\")"=w179) -> ("States Out"=w178:string)  [unwired: 13 in]
          }
          event "Export": Value Change {
            n76 = event-data() -> ()  [unwired: 1 in, 6 out]
            n77 = call "GetExportFolderPath.vi"("error in (no error)"=w190, "DisplayWaveforms"=w192) -> ("error out"=w186:errorcluster, "Export File Folder"=w188:path, "DisplayWaveforms out"=w191:refnum<class "DisplayWaveforms.lvclass">)  [unwired: 7 in]
            n78 = disable-structure shown="Disabled" {
              disable-tunnel: w186 -> [w198 w200]
              disable-tunnel: [w197 w200] -> w185
              frame Disabled {
                # "Also pause chart updates"
                n79 = property on="Update Chart?" class="Bool (strict)"(error in=w198, "Val(Sgnl)"=FALSE ("Value (Signaling)")) -> (error out=w197:errorcluster)  [unwired: 1 in, 1 out]
              }
              frame Enabled {
              }
            }
            n80 = Bundle By Name(cluster=w189, "Export Folder Path"=w188) -> (w187:T47)
            n81 = call "ExportChart.vi"("error in (no error)"=w185, "Export File Folder"=w188, "DisplayWaveforms"=w191) -> ("error out"=w196:errorcluster)  [unwired: 7 in, 1 out]
            n82 = call <vilib>:"Add State(s) to Queue__jki_lib_state_machine.vi"("State(s) in Front (\"\")"="Export: ChartData" ("State(s) in Front (\"\")"), "State(s) in (\"\")"=w194) -> ("States Out"=w193:string)  [unwired: 13 in]
          }
          event "Sequence JSON File Path": Value Change {
            n83 = event-data() -> ()  [unwired: 1 in, 6 out]
            n84 = call <vilib>:"Add State(s) to Queue__jki_lib_state_machine.vi"("State(s) in Front (\"\")"=" PlaMoS: LoadSequence" ("State(s) in Front (\"\")"), "State(s) in (\"\")"=w204) -> ("States Out"=w203:string)  [unwired: 13 in]
          }
          event "Run Plannned Motion Sequence?": Value Change {
            n85 = event-data() -> ("NewVal"=w208:bool)  [unwired: 1 in, 5 out]
            n86 = Bundle By Name(cluster=w210, "UI switch state"=w208) -> (w209:T47)
            n87 = call <vilib>:"Add State(s) to Queue__jki_lib_state_machine.vi"("State(s) in Front (\"\")"="PlaMoS: Start/Stop" ("State(s) in Front (\"\")"), "State(s) in (\"\")"=w211) -> ("States Out"=w212:string)  [unwired: 13 in]
          }
          event "Save\nConfig": Value Change {
            n88 = event-data() -> ()  [unwired: 1 in, 6 out]
            n89 = call <vilib>:"Add State(s) to Queue__jki_lib_state_machine.vi"("State(s) in Front (\"\")"="Config: SaveConfiguration", "State(s) in (\"\")"=w215) -> ("States Out"=w216:string)  [unwired: 13 in]
          }
          event "Load\nConfig": Value Change {
            # "LoadConfiguration file and set zero accordingly"
            n90 = event-data() -> ()  [unwired: 1 in, 6 out]
            n91 = call <vilib>:"Add State(s) to Queue__jki_lib_state_machine.vi"("State(s) in Front (\"\")"="Config: LoadConfiguration\nIP: SetFPGAPosZeroOffset", "State(s) in (\"\")"=w220) -> ("States Out"=w221:string)  [unwired: 13 in]
          }
          event "Run DSA?": Value Change {
            n92 = event-data() -> ("NewVal"=w225:bool)  [unwired: 1 in, 5 out]
            n93 = Bundle By Name(cluster=w227, "UI switch state"=w225) -> (w226:T47)
            n94 = call <vilib>:"Add State(s) to Queue__jki_lib_state_machine.vi"("State(s) in Front (\"\")"="IP: RunDSA" ("State(s) in Front (\"\")"), "State(s) in (\"\")"=w228) -> ("States Out"=w229:string)  [unwired: 13 in]
          }
          event "Export DSA \ndata?": Value Change {
            n95 = event-data() -> ()  [unwired: 1 in, 6 out]
            n96 = call "GetExportFolderPath.vi"("error in (no error)"=w234, "DisplayWaveforms"=w235) -> ("error out"=w230:errorcluster, "Export File Folder"=w232:path)  [unwired: 7 in, 1 out]
            n97 = Bundle By Name(cluster=w233, "Export Folder Path"=w232) -> (w231:T47)
            n98 = call <vilib>:"Add State(s) to Queue__jki_lib_state_machine.vi"("State(s) in Front (\"\")"="Export: DSA Data" ("State(s) in Front (\"\")"), "State(s) in (\"\")"=w237) -> ("States Out"=w236:string)  [unwired: 13 in]
          }
          event "Stop": Value Change {
            # "Stop Communication Process"
            # "Hide UI"
            # "Stop SMO if Stop was pressed"
            # "Exit Button Value Change (pressed) Event\n(this executes Macro: Exit to terminate the VI)"
            n99 = event-data() -> ()  [unwired: 1 in, 6 out]
            n100 = call <vilib>:"Hide.vi"("error in (no error)"=w242, "SMO.UI"=w243) -> ("error out"=w245:errorcluster, "SMO.UI out"=w244:refnum<class "DisplayWaveforms.lvclass">)  [unwired: 8 in]
            n101 = call <vilib>:"Stop.vi"("error in (no error)"=w245, "SMO"=w244) -> ("error out"=w240:errorcluster)  [unwired: 8 in, 1 out]
            n102 = property on="Stop" class="Bool (strict)"(error in=w240, "Value"=FALSE ("Stop")) -> (error out=w239:errorcluster)  [unwired: 1 in, 1 out]
            n103 = call <vilib>:"Add State(s) to Queue__jki_lib_state_machine.vi"("State(s) in Front (\"\")"="Macro: Exit", "State(s) in (\"\")"=w249) -> ("States Out"=w248:string)  [unwired: 13 in]
          }
          event Panel Close? {
            # "Stop SMO if Panel Closed"
            # "Discard the event because we'll close the front panel ourselves in Macro: Exit"
            # "Close Panel button (pressed) Event\n(this executes Macro: Exit to terminate the VI)"
            n104 = event-data() -> ()  [unwired: 1 in, 1 out]
            n105 = call <vilib>:"Hide.vi"("error in (no error)"=w251, "SMO.UI"=w252) -> ("error out"=w253:errorcluster, "SMO.UI out"=w254:refnum<class "DisplayWaveforms.lvclass">)  [unwired: 8 in]
            n106 = call <vilib>:"Stop.vi"("error in (no error)"=w253, "SMO"=w254) -> ("error out"=w250:errorcluster)  [unwired: 8 in, 1 out]
            n107 = event-data("Discard?"=TRUE) -> ()  [unwired: 1 in, 1 out]
            n108 = call <vilib>:"Add State(s) to Queue__jki_lib_state_machine.vi"("State(s) in Front (\"\")"="Macro: Exit", "State(s) in (\"\")"=w259) -> ("States Out"=w258:string)  [unwired: 13 in]
          }
          event User Event {
            n109 = event-data() -> ("SMO State"=w266:T29)  [unwired: 1 in, 4 out]
            n110 = Equal?(x=SMOState_--Enum."Stopped", y=w266) -> (x = y?=w261:bool)
            n111 = case shown="False" w261 {
              tunnel: ["Idle" "Macro: Exit"] -> w260
              frame False {
              }
              frame True {
              }
            }
            n112 = call <vilib>:"Add State(s) to Queue__jki_lib_state_machine.vi"("State(s) in Front (\"\")"=w260, "State(s) in (\"\")"=w263) -> ("States Out"=w262:string)  [unwired: 13 in]
          }
          event User Event {
            # "Stop SMO if UI Closed"
            n113 = event-data() -> ()  [unwired: 1 in, 5 out]
            n114 = call <vilib>:"Stop.vi"("error in (no error)"=w273, "SMO"=w274) -> ("error out"=w272:errorcluster)  [unwired: 8 in, 1 out]
          }
        }
      }
      frame "---------- Core ----------" {
        # "Do not put any code in this frame.\n(it is a separator no-op)"
        n115 = call <vilib>:"Add State(s) to Queue__jki_lib_state_machine.vi"("State(s) in (\"\")"=w278) -> ("States Out"=w277:string)  [unwired: 14 in]
      }
      frame Default {
        w288 = 42 items=["No error", "Argument error", "Memory is full", "Out of zone", "End of file", "File already open", "Generic file I/O error", "File not found", "File permission error", "Disk is full", "Duplicate path", "Too many files open", "System feature not enabled", "Resource file not found", "Cannot add resource", "Resource not found", "Image not found", "Image memory error", "Pen does not exist", "Config type invalid", "Config token not found", "Config parse error", "Config memory error", "Bad external code format", "Bad external code offset", "External code not present", "Null window", "Destroy window error", "Null menu", "Print aborted", "Bad print record", "Print driver error", "Windows error during printing", "Memory error during printing", "Print dialog error", "Generic print error", "Invalid device refnum", "Device not found", "Device parameter error", "Device unit error", "Cannot open device", "Device call aborted", "Generic error", "Cancelled by user", "Object ID too low", "Object ID too high", "Object not in heap", "Unknown heap", "Unknown object (invalid DefProc)", "Unknown object (DefProc not in table)", "Message out of range", "Invalid (null) method", "Unknown message", "Manager call not supported", "Bad address", "Network operation in progress", "Network operation timed out", "Connection is busy", "Network attribute not supported", "Network error", "Address in use", "System out of memory", "Connection aborted", "Connection refused", "Not connected", "Already connected", "Connection closed", "Initialization error (interapplication manager)", "Bad occurrence", "Wait on unbound occurrence handler", "Occurrence queue overflow", "Datalog type conflict", "Unused", "Unrecognized type (interapplication manager)", "Memory corrupt", "Failed to make temporary DLL", "Old CIN version", "Drag socket not found", "Failed to load drop-object", "Failed to register OLE object", "Failed to release OLE object", "Format specifier type mismatch", "Unknown format specifier", "Too few format specifiers", "Too many format specifiers", "Scan failed", "Newer CIN version", "Error converting to variant", "Runtime menu error", "Password tampered", "Variant attribute not found", "Incompatible variant data type", "Event data is not available", "Event Store is not present", "Occurrence is not found", "Event Queue is not created", "Event info is not available", "Refnum passed is NULL", "Error retrieving Class GUID", "Error retrieving CoClass GUID", "Error retrieving TypeLib GUID.", "Bad built application magic bytes.", "Specific driver is different from the specific driver associated with the Logical Name.", "There is no session opened to the class driver.", "Max Error", "MAX - Error with config objects", "MAX - Error loading configuration", "MAX - Group not supported"]
        # "Current State"
        # "Do not delete, rename, or modify this frame.\n(this is used to capture unhandled states and typos)"
        # "Handle mistyped state name (developer tool)"
        n116 = Format Into String(format string="Software Exception: Unhandled State \"%s\"." ("message"), error in=w284, w279) -> (resulting string=w287:string, error out=w286:errorcluster)  [unwired: 1 in]
        n117 = call <vilib>:"Error Cluster From Error Code.vi"("show call chain? (False)"=TRUE, "error in (no error)"=w286, "error message (\"\")"=w287, "error code (0)"=w288) -> ("error out"=w285:errorcluster)  [unwired: 5 in]
        n118 = call <vilib>:"Add State(s) to Queue__jki_lib_state_machine.vi"("State(s) in (\"\")"=w283) -> ("States Out"=w282:string)  [unwired: 14 in]
      }
      frame "Initialize Core Data" {
        # "Do not delete, rename, or modify this frame.\n(this is used to determine panel behavior on exit)"
        # "originally closed?"
        # "exe?"
        # "If panel starts closed or is an EXE, then close it when we exit"
        n119 = property class="VI"() -> ("FP.State"=w292:T30)  [unwired: 2 in, 2 out]
        n120 = property class="App"() -> ("App.Kind"=w298:T31)  [unwired: 2 in, 2 out]
        n121 = control-ref of="Current VI Reference"() -> (w293:refnum<vi>)
        n122 = Equal?(x=w292, y=T30."Closed" ("Front Panel Window:State")) -> (x = y?=w290:bool)
        n123 = Equal?(x=w298, y=T31."Run Time System" ("Application:Kind")) -> (x = y?=w296:bool)
        n124 = Or(x=w290, y=w296) -> (x .or. y?=w294:bool)
        n125 = Bundle By Name(cluster=w295, "Core.Current VI Reference"=w293, "Core.Close Panel on Exit?"=w294) -> (w300:T47)
        n126 = call <vilib>:"Add State(s) to Queue__jki_lib_state_machine.vi"("State(s) in (\"\")"=w302) -> ("States Out"=w301:string)  [unwired: 14 in]
      }
      frame "Error Handler" {
        # "Unhandled Error -- Display it"
        # "Handle any errors here.\nYou can also output any states to clean-up after errors occur"
        # "Clear error"
        n127 = Unbundle By Name(w307) -> ("source"=w305:string)
        n128 = call <vilib>:"General Error Handler.vi"("error in (no error)"=w307) -> ()  [unwired: 10 in, 5 out]
        n129 = Concatenate Strings("/*Post Error States\nStatus: Update >> PC Error: ", w305) -> (w303:string)
        n130 = call <vilib>:"Add State(s) to Queue__jki_lib_state_machine.vi"("State(s) in (\"\")"=w304, "State(s) at Back (\"\")"=w303) -> ("States Out"=w310:string)  [unwired: 13 in]
      }
      frame "Exit" {
        # "Do not put any code in this frame.\n(No errors that occur here will be handled.)"
        n131 = call <vilib>:"Add State(s) to Queue__jki_lib_state_machine.vi"("State(s) in (\"\")"=w316) -> ("States Out"=w315:string)  [unwired: 14 in]
      }
      frame "---------- Data ----------" {
        # "Do not put any code in this frame.\n(It is a separator no-op. You can make a copy of this frame to create a new Data frame)"
        n132 = call <vilib>:"Add State(s) to Queue__jki_lib_state_machine.vi"("State(s) in (\"\")"=w320) -> ("States Out"=w319:string)  [unwired: 14 in]
      }
      frame "Data: Initialize" {
        w321 = path ""  # Export Folder Path
        w322 = T49 {"Current VI Reference"=refnum, "Close Panel on Exit?"=FALSE}  # Core
        w323 = FALSE  # UI switch state
        # "Common Booelan for\nstoring state of any \nUI switch"
        # "Common Booelan for\nstoring state of any \nUI switch"
        # "do not delete - used by framework"
        # "Expand Bundle to add new data elements to shift register data."
        # "Add new data here."
        # "Data names and types of shift register data are defined by this bundle."
        # "Initialize the shift-register data, here.\n(data names are defined by what you wire into the bundle function)"
        n133 = Bundle("Core"=w322, "UI switch state"=w323, "Export Folder Path"=w321) -> (w325:T47)  [unwired: 1 in]
        n134 = call <vilib>:"Add State(s) to Queue__jki_lib_state_machine.vi"("State(s) in (\"\")"=w327) -> ("States Out"=w326:string)  [unwired: 14 in]
      }
      frame "Data: Cleanup" {
        # "Cleanup any data and references, here.\n(this is called automatically, by the Macro: Exit)"
        n135 = Unbundle By Name(w328) -> ("Core.Current VI Reference"=w331:refnum<vi>)
        n136 = Close Reference(reference=w331, error in (no error)=w330) -> (error out=w329:errorcluster)
        n137 = call <vilib>:"Add State(s) to Queue__jki_lib_state_machine.vi"("State(s) in (\"\")"=w333) -> ("States Out"=w332:string)  [unwired: 14 in]
      }
      frame "---------- UI ----------" {
        # "Do not put any code in this frame.\n(It is a separator no-op. You can make a copy of this frame to create a new UI frame)"
        n138 = call <vilib>:"Add State(s) to Queue__jki_lib_state_machine.vi"("State(s) in (\"\")"=w337) -> ("States Out"=w336:string)  [unwired: 14 in]
      }
      frame "UI: Initialize" {
        # "Initialize the User Interface, here.\n(this is called automatically, by the Macro: Init)"
        n139 = disable-structure shown="Enabled" {
          disable-tunnel: w340 -> [w347 _]
          disable-tunnel: [w346 _] -> w339
          frame Enabled {
            # "Reset All front panel controls"
            n140 = control-ref of="This VI"() -> (w348:refnum<vi>)
            n141 = invoke class="VI" method="Default Vals.Reinit All"(reference=w348, error in=w347) -> (error out=w346:errorcluster)  [unwired: 1 in, 2 out]
          }
          frame Disabled {
          }
        }
        n142 = property on="Update Chart?" class="Bool (strict)"(error in=w339, "Val(Sgnl)"=TRUE ("Value (Signaling)")) -> (error out=w338:errorcluster)  [unwired: 1 in, 1 out]
        n143 = call <vilib>:"Add State(s) to Queue__jki_lib_state_machine.vi"("State(s) in Front (\"\")"="Status: Update >> UI Initialized" ("State(s) in Front (\"\")"), "State(s) in (\"\")"=w345) -> ("States Out"=w344:string)  [unwired: 13 in]
      }
      frame "UI: Cursor Set" {
        # "Argument"
        # "Set and Unset Cursor Busy.\n(Usage: \"UI: Cursor Set >> Busy|Idle\")"
        n144 = case shown="\"Idle\", Default" w349 {
          tunnel: w351 -> [w356 w358]
          tunnel: [w355 w357] -> w350
          frame "Idle", Default {
            n145 = call <vilib>:"Unset Busy.vi"("error in (no error)"=w356) -> ("error out"=w355:errorcluster)  [unwired: 10 in]
          }
          frame "Busy" {
            n146 = call <vilib>:"Set Busy.vi"("error in (no error)"=w358) -> ("error out"=w357:errorcluster)  [unwired: 9 in, 1 out]
          }
        }
        n147 = call <vilib>:"Add State(s) to Queue__jki_lib_state_machine.vi"("State(s) in (\"\")"=w354) -> ("States Out"=w353:string)  [unwired: 14 in]
      }
      frame "UI: Front Panel State" {
        # "Argument"
        # "Set Front Panel Open or Closed\n(Usage: \"UI: Front Panel State >> Open|Close\")"
        n148 = Unbundle By Name(w361) -> ("Core.Current VI Reference"=w360:refnum<vi>)
        n149 = case shown="\"Open\", \"Standard\", Default" w359 {
          tunnel: w363 -> [w371 w386 w397 w410 w423]
          tunnel: [w373 w387 w399 w412 w425] -> w362
          tunnel: w360 -> [w372 w384 w398 w411 w424]
          frame "Open", "Standard", Default {
            w366 = T30."Standard" ("State")
            n150 = property class="VI"(reference=w372, error in=w371) -> (reference out=w369:refnum<vi>, error out=w370:errorcluster, "FP.State"=w368:T30)
            n151 = Not Equal?(x=w368, y=w366) -> (x != y?=w367:bool)
            n152 = case shown="False" w367 {
              tunnel: [w377 w379] -> w373
              tunnel: w370 -> [w376 w379]
              tunnel: w369 -> [w375 _]
              tunnel: w366 -> [w374 _]
              frame True {
                n153 = invoke class="VI" method="FP.Open"(reference=w375, error in=w376, "Activate"=TRUE, "State"=w374) -> (error out=w377:errorcluster)  [unwired: 1 in, 4 out]
              }
              frame False {
              }
            }
          }
          frame "Close", "Closed" {
            n154 = property class="VI"(reference=w384, error in=w386) -> (reference out=w383:refnum<vi>, error out=w385:errorcluster, "FP.State"=w381:T30)
            n155 = Not Equal?(x=w381, y=T30."Closed" ("Front Panel Window:State")) -> (x != y?=w380:bool)
            n156 = case shown="True" w380 {
              tunnel: [w388 w391] -> w387
              tunnel: w385 -> [w388 w390]
              tunnel: w383 -> [_ w389]
              frame False {
              }
              frame True {
                n157 = invoke class="VI" method="FP.Close"(reference=w389, error in=w390) -> (error out=w391:errorcluster)  [unwired: 1 in, 2 out]
              }
            }
          }
          frame "Hidden", "Hide" {
            w392 = T30."Hidden" ("State")
            n158 = property class="VI"(reference=w398, error in=w397) -> (reference out=w395:refnum<vi>, error out=w396:errorcluster, "FP.State"=w394:T30)
            n159 = Not Equal?(x=w394, y=w392) -> (x != y?=w393:bool)
            n160 = case shown="True" w393 {
              tunnel: [w403 w404] -> w399
              tunnel: w396 -> [w402 w404]
              tunnel: w395 -> [w401 _]
              tunnel: w392 -> [w400 _]
              frame True {
                n161 = invoke class="VI" method="FP.Open"(reference=w401, error in=w402, "State"=w400) -> (error out=w403:errorcluster)  [unwired: 2 in, 4 out]
              }
              frame False {
              }
            }
          }
          frame "Minimize", "Minimized" {
            w405 = T30."Minimized" ("State")
            n162 = property class="VI"(reference=w411, error in=w410) -> (reference out=w408:refnum<vi>, error out=w409:errorcluster, "FP.State"=w407:T30)
            n163 = Not Equal?(x=w407, y=w405) -> (x != y?=w406:bool)
            n164 = case shown="True" w406 {
              tunnel: [w416 w417] -> w412
              tunnel: w409 -> [w415 w417]
              tunnel: w408 -> [w414 _]
              tunnel: w405 -> [w413 _]
              frame True {
                n165 = invoke class="VI" method="FP.Open"(reference=w414, error in=w415, "State"=w413) -> (error out=w416:errorcluster)  [unwired: 2 in, 4 out]
              }
              frame False {
              }
            }
          }
          frame "Maximize", "Maximized" {
            w418 = T30."Maximized" ("State")
            n166 = property class="VI"(reference=w424, error in=w423) -> (reference out=w421:refnum<vi>, error out=w422:errorcluster, "FP.State"=w420:T30)
            n167 = Not Equal?(x=w420, y=w418) -> (x != y?=w419:bool)
            n168 = case shown="True" w419 {
              tunnel: [w429 w430] -> w425
              tunnel: w422 -> [w428 w430]
              tunnel: w421 -> [w427 _]
              tunnel: w418 -> [w426 _]
              frame True {
                n169 = invoke class="VI" method="FP.Open"(reference=w427, error in=w428, "State"=w426) -> (error out=w429:errorcluster)  [unwired: 2 in, 4 out]
              }
              frame False {
              }
            }
          }
        }
        n170 = call <vilib>:"Add State(s) to Queue__jki_lib_state_machine.vi"("State(s) in (\"\")"=w365) -> ("States Out"=w364:string)  [unwired: 14 in]
      }
      frame "---------- IP ----------" {
        # "Code for inter-process communication \nUse this to send messages via STM to RT target"
        # "Do not put any code in this frame.\n(It is a separator no-op. You can make a copy of this frame to create a new UI frame)"
        n171 = call <vilib>:"Add State(s) to Queue__jki_lib_state_machine.vi"("State(s) in (\"\")"=w434) -> ("States Out"=w433:string)  [unwired: 14 in]
      }
      frame "IP: ReadFPGActrl_loopTime" {
        # "Do not put any code in this frame.\n(It is a separator no-op. You can make a copy of this frame to create a new UI frame)"
        n172 = Bundle By Name(cluster=T32 {"Command"="", "Data"=variant} ("InterProcessQueue"), "Command"="IP: ReadFPGActrl_loopTime") -> (w440:T32)
        n173 = Enqueue Element(queue=w438, element=w440, error in (no error)=w436) -> (error out=w435:errorcluster)  [unwired: 1 in, 2 out]
        n174 = call <vilib>:"Add State(s) to Queue__jki_lib_state_machine.vi"("State(s) in (\"\")"=w443) -> ("States Out"=w442:string)  [unwired: 14 in]
      }
      frame "IP: SetRTtimedLoop_dt" {
        # "During Initialization, Set RT Display Timed Loop Rate"
        # "Do not put any code in this frame.\n(It is a separator no-op. You can make a copy of this frame to create a new UI frame)"
        n175 = local read "RT Display Reader Loop Time [us]"() -> (w444:T15)
        n176 = To Quad Integer(1:w444) -> (0:w448:T15)
        n177 = To Variant(anything=w448) -> (Variant=w449:variant)
        n178 = Bundle By Name(cluster=T32 {"Command"="", "Data"=variant} ("InterProcessQueue"), "Command"="IP: SetRTtimedLoop_dt", "Data"=w449) -> (w451:T32)
        n179 = Enqueue Element(queue=w447, element=w451, error in (no error)=w446) -> (error out=w445:errorcluster)  [unwired: 1 in, 2 out]
        n180 = call <vilib>:"Add State(s) to Queue__jki_lib_state_machine.vi"("State(s) in (\"\")"=w455) -> ("States Out"=w454:string)  [unwired: 14 in]
      }
      frame "IP: AOenable" {
        # "Do not put any code in this frame.\n(It is a separator no-op. You can make a copy of this frame to create a new UI frame)"
        n181 = Unbundle By Name(w460) -> ("UI switch state"=w458:bool)
        n182 = To Variant(anything=w458) -> (Variant=w464:variant)
        n183 = Bundle By Name(cluster=T32 {"Command"="", "Data"=variant} ("InterProcessQueue"), "Command"="IP: AOenable", "Data"=w464) -> (w466:T32)
        n184 = Enqueue Element(queue=w461, element=w466, error in (no error)=w457) -> (error out=w456:errorcluster)  [unwired: 1 in, 2 out]
        n185 = Select(t="Status: Update >> AO enabled" ("State(s) in Front (\"\")"), s=w458, f="Status: Update >> AO disabled" ("State(s) in Front (\"\")")) -> (s? t:f=w459:string)
        n186 = call <vilib>:"Add State(s) to Queue__jki_lib_state_machine.vi"("State(s) in Front (\"\")"=w459, "State(s) in (\"\")"=w469) -> ("States Out"=w468:string)  [unwired: 13 in]
      }
      frame "IP: RunController" {
        # "Do not put any code in this frame.\n(It is a separator no-op. You can make a copy of this frame to create a new UI frame)"
        n187 = Unbundle By Name(w471) -> ("UI switch state"=w470:bool)
        n188 = To Variant(anything=w470) -> (Variant=w481:variant)
        n189 = Bundle By Name(cluster=T32 {"Command"="", "Data"=variant} ("InterProcessQueue"), "Command"="IP: RunCtrl", "Data"=w481) -> (w480:T32)
        n190 = Enqueue Element(queue=w475, element=w480, error in (no error)=w474) -> (error out=w473:errorcluster)  [unwired: 1 in, 2 out]
        n191 = Select(t="Status: Update >> Controller enabled" ("State(s) in Front (\"\")"), s=w470, f="Status: Update >> Controller disabled" ("State(s) in Front (\"\")")) -> (s? t:f=w472:string)
        n192 = call <vilib>:"Add State(s) to Queue__jki_lib_state_machine.vi"("State(s) in Front (\"\")"=w472, "State(s) in (\"\")"=w483) -> ("States Out"=w482:string)  [unwired: 13 in]
      }
      frame "IP: ResetZeroPosition" {
        # "Do not put any code in this frame.\n(It is a separator no-op. You can make a copy of this frame to create a new UI frame)"
        n193 = Bundle By Name(cluster=T32 {"Command"="", "Data"=variant} ("InterProcessQueue"), "Command"="IP: ResetZeroPosition") -> (w489:T32)
        n194 = Enqueue Element(queue=w485, element=w489, error in (no error)=w486) -> (error out=w487:errorcluster)  [unwired: 1 in, 2 out]
        n195 = call <vilib>:"Add State(s) to Queue__jki_lib_state_machine.vi"("State(s) in Front (\"\")"="Status: Update >> Position Zero Offsets updated" ("State(s) in Front (\"\")"), "State(s) in (\"\")"=w493) -> ("States Out"=w492:string)  [unwired: 13 in]
      }
      frame "IP: ViewRawPosition" {
        # "Do not put any code in this frame.\n(It is a separator no-op. You can make a copy of this frame to create a new UI frame)"
        n196 = Bundle By Name(cluster=T32 {"Command"="", "Data"=variant} ("InterProcessQueue"), "Command"="IP: ViewRawPosition") -> (w499:T32)
        n197 = Enqueue Element(queue=w495, element=w499, error in (no error)=w496) -> (error out=w497:errorcluster)  [unwired: 1 in, 2 out]
        n198 = call <vilib>:"Add State(s) to Queue__jki_lib_state_machine.vi"("State(s) in Front (\"\")"="Status: Update >> Position Offsets removed - viewing raw signals" ("State(s) in Front (\"\")"), "State(s) in (\"\")"=w503) -> ("States Out"=w502:string)  [unwired: 13 in]
      }
      frame "IP: ResetZeroCurrSense" {
        # "Do not put any code in this frame.\n(It is a separator no-op. You can make a copy of this frame to create a new UI frame)"
        n199 = Bundle By Name(cluster=T32 {"Command"="", "Data"=variant} ("InterProcessQueue"), "Command"="IP: ResetZeroCurrSense") -> (w509:T32)
        n200 = Enqueue Element(queue=w505, element=w509, error in (no error)=w506) -> (error out=w507:errorcluster)  [unwired: 1 in, 2 out]
        n201 = call <vilib>:"Add State(s) to Queue__jki_lib_state_machine.vi"("State(s) in Front (\"\")"="Status: Update >> Current Sense Zero Offsets updated" ("State(s) in Front (\"\")"), "State(s) in (\"\")"=w513) -> ("States Out"=w512:string)  [unwired: 13 in]
      }
      frame "IP: UpdateCtrlGains" {
        # "Do not put any code in this frame.\n(It is a separator no-op. You can make a copy of this frame to create a new UI frame)"
        n202 = To Variant(anything="Controller Gains") -> (Variant=w519:variant)
        n203 = Bundle By Name(cluster=T32 {"Command"="", "Data"=variant} ("InterProcessQueue"), "Command"="IP: UpdateCtrlParams", "Data"=w519) -> (w521:T32)
        n204 = Enqueue Element(queue=w518, element=w521, error in (no error)=w517) -> (error out=w516:errorcluster)  [unwired: 1 in, 2 out]
        n205 = call <vilib>:"Add State(s) to Queue__jki_lib_state_machine.vi"("State(s) in Front (\"\")"="Status: Update >> Controller Gains Updated" ("State(s) in Front (\"\")"), "State(s) in (\"\")"=w525) -> ("States Out"=w524:string)  [unwired: 13 in]
      }
      frame "IP: SetFPGAPosZeroOffset" {
        # "Do not put any code in this frame.\n(It is a separator no-op. You can make a copy of this frame to create a new UI frame)"
        n206 = To Variant(anything="Pos Zero Offsets [V]") -> (Variant=w531:variant)
        n207 = Bundle By Name(cluster=T32 {"Command"="", "Data"=variant} ("InterProcessQueue"), "Command"="IP: SetFPGAPosZeroOffset", "Data"=w531) -> (w533:T32)
        n208 = Enqueue Element(queue=w530, element=w533, error in (no error)=w529) -> (error out=w528:errorcluster)  [unwired: 1 in, 2 out]
        n209 = call <vilib>:"Add State(s) to Queue__jki_lib_state_machine.vi"("State(s) in Front (\"\")"="Status: Update >> FPGA PosMeas ZeroOffset values set. " ("State(s) in Front (\"\")"), "State(s) in (\"\")"=w537) -> ("States Out"=w536:string)  [unwired: 13 in]
      }
      frame "IP: UpdateReference" {
        # "Convert Frequency from\nHz to periods per tick"
        # "Do not put any code in this frame.\n(It is a separator no-op. You can make a copy of this frame to create a new UI frame)"
        n210 = Unbundle By Name("Reference Generation") -> ("Reference Location"=w551:T5, "Direction"=w550:enum16{"Z", "ThX", "ThY", "Bow", "B-d"}, "Excitation Mode"=w549:enum16{"DC", "Sine", "Square", "WhiteNoise"}, "Amplitude"=w548:dbl, "Frequency [Hz]"=w547:dbl, "PosRef Offsets"=w544:T6)
        n211 = Cluster To Array(cluster=w544) -> (array=w543:dbl[])
        n212 = Multiply(x=w547, y=2.5e-08) -> (x*y=w545:dbl)
        n213 = Bundle By Name(cluster=T33 {"Reference Location"=enum."Pos Ref", "Direction"=enum."Z", "Excitation mode"=enum."DC", "Amplitude"=0.0, "Frequency (periods/tick)"=0.0, "PosRef_Offset"=[]} ("FuncGen Params"), "Reference Location"=w551, "Direction"=w550, "Excitation mode"=w549, "Amplitude"=w548, "Frequency (periods/tick)"=w545, "PosRef_Offset"=w543) -> (w553:T33)
        n214 = To Variant(anything=w553) -> (Variant=w554:variant)
        n215 = Bundle By Name(cluster=T32 {"Command"="", "Data"=variant} ("InterProcessQueue"), "Command"="IP: UpdateReference", "Data"=w554) -> (w556:T32)
        n216 = Enqueue Element(queue=w542, element=w556, error in (no error)=w540) -> (error out=w539:errorcluster)  [unwired: 1 in, 2 out]
        n217 = call <vilib>:"Add State(s) to Queue__jki_lib_state_machine.vi"("State(s) in Front (\"\")"="Status: Update >> Reference Params Updated" ("State(s) in Front (\"\")"), "State(s) in (\"\")"=w560) -> ("States Out"=w559:string)  [unwired: 13 in]
      }
      frame "IP: RunDSA" {
        # "#MAYBE: Split into two cases - StartDSA and Stop DSA\nand call those two cases from this case."
        # "Do not put any code in this frame.\n(It is a separator no-op. You can make a copy of this frame to create a new UI frame)"
        n218 = Unbundle By Name(w571) -> ("UI switch state"=w567:bool)
        n219 = control-ref of="DSA excitation specs"() -> (w563:refnum<vi>)
        n220 = control-ref of="Cycle Specs"() -> (w564:refnum<vi>)
        n221 = Build Array(w563, w564) -> (w562:refnum<vi>[])
        n222 = case shown="False" w567 {
          tunnel: [w580 w592] -> w575
          tunnel: "Cycle Specs" -> [_ w587]
          tunnel: "DSA excitation specs" -> [_ w586]
          tunnel: w562 -> [w578 w585]
          tunnel: "Meas. TF params" -> [_ w584]
          frame False {
            n223 = for {
              tunnel: w578 -> [w583] mode=indexing
              n224 = property class="Clust"(reference=w583, "DisabledEnum"=T35."Enabled" ("Disabled")) -> ()  [unwired: 1 in, 2 out]
            }
            n225 = Bundle By Name(cluster=T32 {"Command"="", "Data"=variant} ("InterProcessQueue"), "Command"="IP: StopDSA") -> (w580:T32)
          }
          frame True {
            n226 = Bundle By Name(cluster=T36 {"DSA excitation specs"={"Initial Freq. [Hz]"=1.0, "Final Freq. [Hz]"=100.0, "# pts. in interval"=20, "Samping Time [us]"=0.0, "Amplitude"=0.0003, "Offset [V]"=0.0, "Freq Units (F: rad/s, T: Hz)"=TRUE}, "Cycle Specs"={"Cycles To \nSettle (M)"=1, "Cycles To \nCalculate (N)"=2}, "Meas. TF params"={"Direction"=enum."Z", "Tras. Func."=enum."P"}} ("DSA Config Cluster"), "DSA excitation specs"=w586, "Cycle Specs"=w587, "Meas. TF params"=w584) -> (w589:T36)
            n227 = for {
              tunnel: w585 -> [w595] mode=indexing
              n228 = property class="Clust"(reference=w595, "DisabledEnum"=T35."Disabled and Grayed Out" ("Disabled")) -> ()  [unwired: 1 in, 2 out]
            }
            n229 = To Variant(anything=w589) -> (Variant=w590:variant)
            n230 = Bundle By Name(cluster=T32 {"Command"="", "Data"=variant} ("InterProcessQueue"), "Command"="IP: StartDSA", "Data"=w590) -> (w592:T32)
          }
        }
        n231 = Select(t="Status: Update >>DSA Running" ("State(s) in Front (\"\")"), s=w567, f="Status: Update >>DSA Stopped" ("State(s) in Front (\"\")")) -> (s? t:f=w569:string)
        n232 = Enqueue Element(queue=w574, element=w575, error in (no error)=w573) -> (error out=w572:errorcluster)  [unwired: 1 in, 2 out]
        n233 = call <vilib>:"Add State(s) to Queue__jki_lib_state_machine.vi"("State(s) in Front (\"\")"=w569, "State(s) in (\"\")"=w577) -> ("States Out"=w576:string)  [unwired: 13 in]
      }
      frame "---------- Macro ----------" {
        # "Do not put any code in this frame.\n(It is a separator no-op. You can make a copy of this frame to create a new Macro frame)"
        n234 = call <vilib>:"Add State(s) to Queue__jki_lib_state_machine.vi"("State(s) in (\"\")"=w599) -> ("States Out"=w598:string)  [unwired: 14 in]
      }
      frame "Macro: Initialize" {
        # "Initialization Macro\n(This is called once, when the VI starts)"
        n235 = call <vilib>:"Add State(s) to Queue__jki_lib_state_machine.vi"("State(s) in Front (\"\")"="Data: Initialize\nInitialize Core Data\n// UI\nUI: Initialize\nUI: Front Panel State >> Open\n// Config\nConfig: LoadConfiguration\nConfig: SendGraphConfig\n// IP\nIP: SetRTtimedLoop_dt \nIP: ReadFPGActrl_loopTime\nIP: SetFPGAPosZeroOffset\nIP: UpdateCtrlGains\nIP: UpdateReference\nIP: RunDSA\n// Status\nStatus: Update >> Controller Initialized", "State(s) in (\"\")"=w604) -> ("States Out"=w603:string)  [unwired: 13 in]
      }
      frame "Macro: Exit" {
        # "Tell RT Target to ShutDown"
        # "Set Stop Global Variable to True"
        # "Exit Macro\n(This is called once, when the VI exits)"
        n236 = Unbundle By Name(w619) -> ("Core.Close Panel on Exit?"=w618:bool)
        n237 = Bundle By Name(cluster=T32 {"Command"="", "Data"=variant} ("InterProcessQueue"), "Command"="IP: ShutDown") -> (w610:T32)
        n238 = Enqueue Element(queue=w605, element=w610, error in (no error)=w608) -> (error out=w607:errorcluster)  [unwired: 1 in, 2 out]
        n239 = shared-variable ".\\Variables.lvlib\\Stop"(TRUE ("Stop"), error in=w607) -> (error out=w606:errorcluster)
        n240 = Select(t="UI: Front Panel State >> Close", s=w618, f="") -> (s? t:f=w615:string)
        n241 = call <vilib>:"Add State(s) to Queue__jki_lib_state_machine.vi"("State(s) in (\"\")"=w615, "State(s) at Back (\"\")"="Data: Cleanup\nPlaMoS: StopSequence\nConfig: SaveConfiguration\nStatus: Update >> Exiting Program\nExit") -> ("States Out"=w613:string)  [unwired: 13 in]
        n242 = call <vilib>:"Add State(s) to Queue__jki_lib_state_machine.vi"("State(s) in Front (\"\")"=w613, "State(s) in (\"\")"=w621) -> ("States Out"=w620:string)  [unwired: 13 in]
      }
      frame "---------- Config ----------" {
        # "Template Separator\n(You can make a copy of, or modify, this frame)"
        n243 = call <vilib>:"Add State(s) to Queue__jki_lib_state_machine.vi"("State(s) in (\"\")"=w625) -> ("States Out"=w624:string)  [unwired: 14 in]
      }
      frame "Config: LoadConfiguration" {
        # "Read \nentire\nfile"
        # "Template Separator\n(You can make a copy of, or modify, this frame)"
        n244 = call <vilib>:"Application Directory.vi"() -> ("Application Directory"=w658:path)
        n245 = Build Path(base path=w658, name or relative path=path "Config.json") -> (appended path=w656:path)
        n246 = Open/Create/Replace File(file path (use dialog)=w656, error in=w654, operation (0:open)=T38."open") -> (refnum out=w651:refnum<file>, error out=w652:errorcluster)  [unwired: 3 in, 1 out]
        n247 = Read from Binary File(8:w652, 10:-1 ("count (1)"), 11:w651) -> (0:w647:errorcluster, 2:w648:string, 3:w650:refnum<file>)  [unwired: 3 in, 1 out]
        n248 = call <vilib>:"Reformat.vi"("Pretty Print Levels"=0, "error in (no error)"=w647, "JSON"=w648) -> ("error out"=w646:errorcluster, "<JSON>"=w649:string)  [unwired: 5 in, 2 out]
        n249 = call "From JSON Text.vim"("Data Type and Default Value"=T37 {"Controller Gains"={"Z-direction"={"Kp"=0.0, "Ki"=0.0, "fLPF"=0.0}, "ThX-direction"={"Kp"=0.0, "Ki"=0.0, "fLPF"=0.0}, "ThY-direction"={"Kp"=0.0, "Ki"=0.0, "fLPF"=0.0}, "Bow-direction"={"Kp"=0.0, "Ki"=0.0, "fLPF"=0.0}, "B-d - direction"={"Kp"=0.0, "Ki"=0.0, "fLPF"=0.0}}, "Reference Generation"={"Reference Location"=enum."Pos Ref", "Direction"=enum."Z", "Excitation Mode"=enum."DC", "Amplitude"=0.0, "Frequency [Hz]"=0.0, "PosRef Offsets"={"Z"=0.0, "ThX"=0.0, "ThY"=0.0, "Bow"=0.0, "B-d"=0.0}, "Inc Offset (PosRef)"={"Step"=0.0, "Arrow Up"=FALSE, "Arrow Down"=FALSE}}, "RT Display Reader Loop Time [us]"=0, "Sensor Gains [um/V]"={"G_SE"=0.0, "G_NE"=0.0, "G_NW"=0.0, "G_SW"=0.0, "G_CI"=0.0}, "Amplifier Gains [V/V]"={"G_SE"=0.0, "G_NE"=0.0, "G_NW"=0.0, "G_SW"=0.0, "G_CO"=0.0, "G_CI"=0.0}, "Curr Sense Gain [mA/V]"={"G_CS"=0.0}, "Sensor Offset  [mm]"={"X"=1.0, "Y"=1.0}, "Coord. Trans. Multipliers"={"Z"=0.0, "Th"=0.0}, "DSA Config Cluster"={"DSA excitation specs"={"Initial Freq. [Hz]"=0.0, "Final Freq. [Hz]"=0.0, "# pts. in interval"=0, "Samping Time [us]"=0.0, "Amplitude"=0.0, "Offset [V]"=0.0, "Freq Units (F: rad/s, T: Hz)"=FALSE}, "Cycle Specs"={"Cycles To \nSettle (M)"=0, "Cycles To \nCalculate (N)"=0}, "Meas. TF params"={"Direction"=enum."Z", "Tras. Func."=enum."P"}}, "Pos Zero Offsets [V]"={"V_SE"=0.0, "V_NE"=0.0, "V_NW"=0.0, "V_SW"=0.0, "V_CI"=0.0}} ("Config Cluster"), "error in (no error)"=w646, "JSON"=w649) -> ("error out"=w633:errorcluster, "Data out"=w641:T37)  [unwired: 7 in]
        n250 = Unbundle By Name(w641) -> ("Controller Gains"=w629:T2, "Reference Generation"=w638:T4, "RT Display Reader Loop Time [us]"=w639:i64, "Sensor Gains [um/V]"=w637:T19, "Amplifier Gains [V/V]"=w636:T18, "Curr Sense Gain [mA/V]"=w635:T16, "Sensor Offset  [mm]"=w632:T14, "Coord. Trans. Multipliers"=w630:T13, "DSA Config Cluster"=w631:T36, "Pos Zero Offsets [V]"=w628:T20)
        n251 = Close File(refnum=w650, error in=w647) -> (error out=w645:errorcluster)  [unwired: 1 out]
        n252 = Merge Errors(w633, w645) -> (w644:errorcluster)
        n253 = Unbundle(w631) -> ("DSA excitation specs"=w634:T12, "Cycle Specs"=w627:T11, "Meas. TF params"=w626:T9)
        n254 = local write "Controller Gains"(w629) -> ()
        n255 = local write "Reference Generation"(w638) -> ()
        n256 = local write "RT Display Reader Loop Time [us]"(w639) -> ()
        n257 = local write "Sensor Gains [um/V]"(w637) -> ()
        n258 = local write "Amplifier Gains [V/V]"(w636) -> ()
        n259 = local write "Curr Sense Gain [mA/V]"(w635) -> ()
        n260 = local write "Sensor H-Offset  [mm]"(w632) -> ()
        n261 = local write "Coord. Trans. Multipliers"(w630) -> ()
        n262 = local write "DSA excitation specs"(w634) -> ()
        n263 = local write "Cycle Specs"(w627) -> ()
        n264 = local write "Meas. TF params"(w626) -> ()
        n265 = local write "Pos Zero Offsets [V]"(w628) -> ()
        n266 = call <vilib>:"Add State(s) to Queue__jki_lib_state_machine.vi"("State(s) in Front (\"\")"="\nStatus: Update >> Params loaded from Config file" ("State(s) in Front (\"\")"), "State(s) in (\"\")"=w661) -> ("States Out"=w660:string)  [unwired: 13 in]
      }
      frame "Config: SaveConfiguration" {
        # "Template Separator\n(You can make a copy of, or modify, this frame)"
        n267 = case shown="\"idle\", Default" w667 {
          tunnel: [w697 w701] -> w694
          tunnel: w666 -> [w700 _]
          frame "Export" {
            # "Use export folder path."
            n268 = Unbundle By Name(w700) -> ("Export Folder Path"=w699:path)
            n269 = Build Path(base path=w699, name or relative path=path "Config.json") -> (appended path=w697:path)
          }
          frame "idle", Default {
            # "Use Config file in project folder"
            n270 = call <vilib>:"Application Directory.vi"() -> ("Application Directory"=w703:path)
            n271 = Build Path(base path=w703, name or relative path=path "Config.json") -> (appended path=w701:path)
          }
        }
        n272 = local read "Controller Gains"() -> (w665:T2)
        n273 = local read "Reference Generation"() -> (w679:T4)
        n274 = local read "RT Display Reader Loop Time [us]"() -> (w678:T15)
        n275 = local read "Sensor Gains [um/V]"() -> (w677:T19)
        n276 = local read "Amplifier Gains [V/V]"() -> (w676:T18)
        n277 = local read "Curr Sense Gain [mA/V]"() -> (w675:T16)
        n278 = local read "Sensor H-Offset  [mm]"() -> (w670:T14)
        n279 = local read "Coord. Trans. Multipliers"() -> (w668:T13)
        n280 = local read "DSA excitation specs"() -> (w674:T12)
        n281 = local read "Cycle Specs"() -> (w673:T11)
        n282 = local read "Meas. TF params"() -> (w664:T9)
        n283 = local read "Pos Zero Offsets [V]"() -> (w663:T20)
        n284 = Bundle(cluster=T36 {"DSA excitation specs"={"Initial Freq. [Hz]"=1.0, "Final Freq. [Hz]"=100.0, "# pts. in interval"=20, "Samping Time [us]"=0.0, "Amplitude"=0.0003, "Offset [V]"=0.0, "Freq Units (F: rad/s, T: Hz)"=TRUE}, "Cycle Specs"={"Cycles To \nSettle (M)"=1, "Cycles To \nCalculate (N)"=2}, "Meas. TF params"={"Direction"=enum."Z", "Tras. Func."=enum."P"}} ("DSA Config Cluster"), "DSA excitation specs"=w674, "Cycle Specs"=w673, "Meas. TF params"=w664) -> (w669:T36)
        n285 = Open/Create/Replace File(file path (use dialog)=w694, error in=w682, operation (0:open)=T38."open or create") -> (refnum out=w687:refnum<file>, error out=w662:errorcluster)  [unwired: 3 in, 1 out]
        n286 = Bundle(cluster=T37 {"Controller Gains"={"Z-direction"={"Kp"=0.0, "Ki"=0.0, "fLPF"=0.0}, "ThX-direction"={"Kp"=0.0, "Ki"=0.0, "fLPF"=0.0}, "ThY-direction"={"Kp"=0.0, "Ki"=0.0, "fLPF"=0.0}, "Bow-direction"={"Kp"=0.0, "Ki"=0.0, "fLPF"=0.0}, "B-d - direction"={"Kp"=0.0, "Ki"=0.0, "fLPF"=0.0}}, "Reference Generation"={"Reference Location"=enum."Pos Ref", "Direction"=enum."Z", "Excitation Mode"=enum."DC", "Amplitude"=0.0, "Frequency [Hz]"=0.0, "PosRef Offsets"={"Z"=0.0, "ThX"=0.0, "ThY"=0.0, "Bow"=0.0, "B-d"=0.0}, "Inc Offset (PosRef)"={"Step"=0.0, "Arrow Up"=FALSE, "Arrow Down"=FALSE}}, "RT Display Reader Loop Time [us]"=0, "Sensor Gains [um/V]"={"G_SE"=0.0, "G_NE"=0.0, "G_NW"=0.0, "G_SW"=0.0, "G_CI"=0.0}, "Amplifier Gains [V/V]"={"G_SE"=0.0, "G_NE"=0.0, "G_NW"=0.0, "G_SW"=0.0, "G_CO"=0.0, "G_CI"=0.0}, "Curr Sense Gain [mA/V]"={"G_CS"=0.0}, "Sensor Offset  [mm]"={"X"=1.0, "Y"=1.0}, "Coord. Trans. Multipliers"={"Z"=0.0, "Th"=0.0}, "DSA Config Cluster"={"DSA excitation specs"={"Initial Freq. [Hz]"=0.0, "Final Freq. [Hz]"=0.0, "# pts. in interval"=0, "Samping Time [us]"=0.0, "Amplitude"=0.0, "Offset [V]"=0.0, "Freq Units (F: rad/s, T: Hz)"=FALSE}, "Cycle Specs"={"Cycles To \nSettle (M)"=0, "Cycles To \nCalculate (N)"=0}, "Meas. TF params"={"Direction"=enum."Z", "Tras. Func."=enum."P"}}, "Pos Zero Offsets [V]"={"V_SE"=0.0, "V_NE"=0.0, "V_NW"=0.0, "V_SW"=0.0, "V_CI"=0.0}} ("output cluster"), "Controller Gains"=w665, "Reference Generation"=w679, "RT Display Reader Loop Time [us]"=w678, "Sensor Gains [um/V]"=w677, "Amplifier Gains [V/V]"=w676, "Curr Sense Gain [mA/V]"=w675, "Sensor Offset  [mm]"=w670, "Coord. Trans. Multipliers"=w668, "DSA Config Cluster"=w669, "Pos Zero Offsets [V]"=w663) -> (w680:T37)
        n287 = call "To JSON Text.vim"("error in (no error)"=w662, "Anything"=w680) -> ("error out"=w685:errorcluster, "<JSON>"=w689:string)  [unwired: 8 in]
        n288 = call <vilib>:"Reformat.vi"("Pretty Print Levels"=10, "error in (no error)"=w685, "JSON"=w689) -> ("error out"=w684:errorcluster, "<JSON>"=w686:string)  [unwired: 5 in, 2 out]
        n289 = Merge Errors(w684, w662) -> (w683:errorcluster)
        n290 = Write to Text File(file (use dialog)=w687, text=w686, error in=w683) -> (refnum out=w692:refnum<file>, error out=w691:errorcluster)  [unwired: 1 in, 1 out]
        n291 = Close File(refnum=w692, error in=w691) -> (error out=w681:errorcluster)  [unwired: 1 out]
        n292 = call <vilib>:"Add State(s) to Queue__jki_lib_state_machine.vi"("State(s) in Front (\"\")"="Status: Update >> Config File Updated" ("State(s) in Front (\"\")"), "State(s) in (\"\")"=w696) -> ("States Out"=w695:string)  [unwired: 13 in]
      }
      frame "Config: SendGraphConfig" {
        # "Send scaling parameters to graph to plot values correctly."
        # "Update Coord. Transform multipliers"
        n293 = Bundle By Name(cluster=T39 {"RT Display Reader Loop Time [us]"=1000, "Sensor Gains [um/V]"={"G_SE"=1.0, "G_NE"=1.0, "G_NW"=1.0, "G_SW"=1.0, "G_CI"=1.0}, "Sensor H-Offset  [mm]"={"X"=1.0, "Y"=1.0}, "Amplifier Gains [V/V]"={"G_SE"=1.0, "G_NE"=1.0, "G_NW"=1.0, "G_SW"=1.0, "G_CO"=1.0, "G_CI"=1.0}, "Curr Sense Gain [mA/V]"={"G_CS"=0.0}} ("GraphInfoCluster"), "RT Display Reader Loop Time [us]"="RT Display Reader Loop Time [us]", "Sensor Gains [um/V]"="Sensor Gains [um/V]", "Sensor H-Offset  [mm]"="Sensor H-Offset  [mm]", "Amplifier Gains [V/V]"="Amplifier Gains [V/V]", "Curr Sense Gain [mA/V]"="Curr Sense Gain [mA/V]") -> (w711:T39)
        n294 = call "GetChartParams.vi"("error in (no error)"=w714, "GraphInfoCluster"=w711, "DisplayWaveforms"=w717) -> ("error out"=w715:errorcluster, "ChartParams"=w706:T50, "DisplayWaveforms out"=w716:refnum<class "DisplayWaveforms.lvclass">)  [unwired: 6 in]
        n295 = Unbundle By Name(w706) -> ("Coord Transform Multipliers"=w705:cluster{"Z-Multiplier":dbl, "Th-Multiplier":dbl})
        n296 = call "SetChartParams.vi"("error in (no error)"=w715, "ChartParams"=w706, "DisplayWaveforms"=w716) -> ("error out"=w713:errorcluster)  [unwired: 7 in, 1 out]
        n297 = local write "Coord. Trans. Multipliers"(w705) -> ()
        n298 = call <vilib>:"Add State(s) to Queue__jki_lib_state_machine.vi"("State(s) in Front (\"\")"="Status: Update >> Chart Params Updated" ("State(s) in Front (\"\")"), "State(s) in (\"\")"=w718) -> ("States Out"=w719:string)  [unwired: 13 in]
      }
      frame "---------- Status ----------" {
        # "Template Separator\n(You can make a copy of, or modify, this frame)"
        n299 = call <vilib>:"Add State(s) to Queue__jki_lib_state_machine.vi"("State(s) in (\"\")"=w725) -> ("States Out"=w724:string)  [unwired: 14 in]
      }
      frame "Status: Update" {
        # "Display first current and previous status update."
        # "Template Separator\n(You can make a copy of, or modify, this frame)"
        n300 = feedback-in #1(w726) -> ()
        n301 = feedback #1() -> (w727:string)  [unwired: 1 in]
        n302 = Concatenate Strings("Prev: " ("string"), w727, "\nCurr: " ("string"), w726) -> (→"Status":string)
        n303 = call <vilib>:"Add State(s) to Queue__jki_lib_state_machine.vi"("State(s) in (\"\")"=w734) -> ("States Out"=w733:string)  [unwired: 14 in]
      }
      frame "---------- Export ----------" {
        # "Template Separator\n(You can make a copy of, or modify, this frame)"
        n304 = call <vilib>:"Add State(s) to Queue__jki_lib_state_machine.vi"("State(s) in (\"\")"=w738) -> ("States Out"=w737:string)  [unwired: 14 in]
      }
      frame "Export: ChartData" {
        # "Template Separator\n(You can make a copy of, or modify, this frame)"
        n305 = call <vilib>:"Add State(s) to Queue__jki_lib_state_machine.vi"("State(s) in Front (\"\")"="Config: SaveConfiguration >> Export\nStatus: Update >> Charts Exported" ("State(s) in Front (\"\")"), "State(s) in (\"\")"=w743) -> ("States Out"=w742:string)  [unwired: 13 in]
      }
      frame "Export: DSA Data" {
        # "Template Separator\n(You can make a copy of, or modify, this frame)"
        n306 = local read "Bode Data"() -> (w756:T8)
        n307 = Unbundle(w756) -> ("Magnitude Bode Plot"=w755:cluster{dbl[], dbl[]}, "Phase Bode Plot"=w754:cluster{dbl[], dbl[]})
        n308 = Unbundle(w755) -> (w753:dbl[], w752:dbl[])
        n309 = Unbundle(w754) -> (w751:dbl[])  [unwired: 1 out]
        n310 = Unbundle By Name(w762) -> ("Export Folder Path"=w757:path)
        n311 = Bundle By Name(cluster=T40 {"Frequency [Hz]"=[], "Magnitude [abs]"=[], "Phase [deg]"=[]} ("Bode Plots"), "Frequency [Hz]"=w753, "Magnitude [abs]"=w752, "Phase [deg]"=w751) -> (w759:T40)
        n312 = call "ExportDSAdata.vi"("error in (no error)"=w761, "Export Folder Path"=w757, "Bode Plots"=w759) -> ("error out"=w750:errorcluster)  [unwired: 8 in]
        n313 = invoke on="Bode Data" class="Clust (strict)" method="Get Image"(error in=w750, "bg color"=u32 16777225 ("Background Color")) -> (error out=w747:errorcluster, "image data"=w749:T51)  [unwired: 4 in, 4 out]
        n314 = Build Path(base path=w757, name or relative path=path "bode.png") -> (appended path=w748:path)
        n315 = call <vilib>:"Write PNG File.vi"("compression (default)"=-1, "error in (no error)"=w747, "image data"=w749, "path to PNG file"=w748) -> ("error out"=w745:errorcluster)  [unwired: 6 in, 1 out]
        n316 = call <vilib>:"Add State(s) to Queue__jki_lib_state_machine.vi"("State(s) in Front (\"\")"="Config: SaveConfiguration >> Export\nStatus: Update >> DSA Data Exported" ("State(s) in Front (\"\")"), "State(s) in (\"\")"=w765) -> ("States Out"=w764:string)  [unwired: 13 in]
      }
      frame "---------- PlaMoS ----------" {
        # "Template Separator\n(You can make a copy of, or modify, this frame)"
        n317 = call <vilib>:"Add State(s) to Queue__jki_lib_state_machine.vi"("State(s) in (\"\")"=w769) -> ("States Out"=w768:string)  [unwired: 14 in]
      }
      frame "PlaMoS: LoadSequence" {
        # "Read \nentire\nfile"
        # "Template Separator\n(You can make a copy of, or modify, this frame)"
        n318 = Open/Create/Replace File(file path (use dialog)="Sequence JSON File Path", error in=w775, operation (0:open)=T38."open") -> (refnum out=w782:refnum<file>, error out=w783:errorcluster)  [unwired: 3 in, 1 out]
        n319 = Read from Binary File(8:w783, 10:-1 ("count (1)"), 11:w782) -> (0:w779:errorcluster, 2:w780:string, 3:w781:refnum<file>)  [unwired: 3 in, 1 out]
        n320 = call <vilib>:"Reformat.vi"("Pretty Print Levels"=20, "error in (no error)"=w779, "JSON"=w780) -> ("error out"=w771:errorcluster, "<JSON>"=→"Loaded Sequence":string)  [unwired: 5 in, 2 out]
        n321 = disable-structure shown="Enabled" {
          disable-tunnel: w771 -> [w794 _]
          frame Enabled {
            # "Create Sample JSON file"
            n322 = call <vilib>:"Application Directory.vi"() -> ("Application Directory"=w800:path)
            n323 = Build Path(base path=w800, name or relative path=path "PlaMoS_seq_sample.json") -> (appended path=w795:path)
            n324 = Open/Create/Replace File(file path (use dialog)=w795, error in=w794, operation (0:open)=T38."open or create") -> (refnum out=w793:refnum<file>, error out=w797:errorcluster)  [unwired: 3 in, 1 out]
            n325 = call "To JSON Text.vim"("Anything"=T41 [{"_Comment"="test", "StepParams"={"Ctrl State"=enum."PosCtrl", "CtrlEff Params"={"Time [s]"=0.0, "U_z"=0.0}, "PosCtrl Params"={"Velocity [um/s]"=0.0, "Starting Z-position [um]"=0.0, "Ending Z-position [um]"=0.0, "Bow Reference [um]"=0.0}, "HoldState Params"={"Time [s]"=0.0}}, "Controller Gains"={"Z-direction"={"Kp"=1.0, "Ki"=0.0, "fLPF"=0.0}, "ThX-direction"={"Kp"=0.0, "Ki"=0.0, "fLPF"=0.0}, "ThY-direction"={"Kp"=0.0, "Ki"=0.0, "fLPF"=0.0}, "Bow-direction"={"Kp"=0.0, "Ki"=0.0, "fLPF"=0.0}, "B-d - direction"={"Kp"=0.0, "Ki"=0.0, "fLPF"=0.0}}}] ("Planned Motion Sequence Steps")) -> ("error out"=w801:errorcluster, "<JSON>"=w803:string)  [unwired: 9 in]
            n326 = call <vilib>:"Reformat.vi"("Pretty Print Levels"=20, "error in (no error)"=w801, "JSON"=w803) -> ("error out"=w792:errorcluster, "<JSON>"=w789:string)  [unwired: 5 in, 2 out]
            n327 = Merge Errors(w792, w797) -> (w796:errorcluster)
            n328 = Write to Text File(file (use dialog)=w793, text=w789, error in=w796) -> (refnum out=w790:refnum<file>, error out=w791:errorcluster)  [unwired: 1 in, 1 out]
            n329 = Close File(refnum=w790, error in=w791) -> ()  [unwired: 2 out]
          }
          frame Disabled {
          }
        }
        n330 = Close File(refnum=w781, error in=w779) -> (error out=w778:errorcluster)  [unwired: 1 out]
        n331 = Merge Errors(w771, w778) -> (w773:errorcluster)
        n332 = call <vilib>:"Add State(s) to Queue__jki_lib_state_machine.vi"("State(s) in Front (\"\")"="Status: Update >> PlaMoS steps loaded" ("State(s) in Front (\"\")"), "State(s) in (\"\")"=w787) -> ("States Out"=w786:string)  [unwired: 13 in]
      }
      frame "PlaMos: Start/Stop" {
        # "Do not put any code in this frame.\n(It is a separator no-op. You can make a copy of this frame to create a new UI frame)"
        n333 = Unbundle By Name(w809) -> ("UI switch state"=w805:bool)
        n334 = Select(t="PlaMoS: StartSequence" ("State(s) in Front (\"\")"), s=w805, f="PlaMoS: StopSequence" ("State(s) in Front (\"\")")) -> (s? t:f=w807:string)
        n335 = call <vilib>:"Add State(s) to Queue__jki_lib_state_machine.vi"("State(s) in Front (\"\")"=w807, "State(s) in (\"\")"=w811) -> ("States Out"=w810:string)  [unwired: 13 in]
      }
      frame "PlaMoS: StartSequence" {
        # "Don't give control during sequence running"
        # "Save current config"
        # "Template Separator\n(You can make a copy of, or modify, this frame)"
        n336 = local read "Loaded Sequence"() -> (w826:string)
        n337 = Empty String/Path?(string/path=w826) -> (empty?=w825:bool)
        n338 = control-ref of="Reference Generation"() -> (w813:refnum<vi>)
        n339 = control-ref of="Update Controller Gains"() -> (w820:refnum<vi>)
        n340 = control-ref of="Update Reference"() -> (w819:refnum<vi>)
        n341 = control-ref of="Zero Curr. Sense"() -> (w818:refnum<vi>)
        n342 = control-ref of="Set Pos. Zero"() -> (w817:refnum<vi>)
        n343 = control-ref of="Run Controller?"() -> (w816:refnum<vi>)
        n344 = control-ref of="Set Pos. Zero"() -> (w815:refnum<vi>)
        n345 = control-ref of="Run DSA?"() -> (w814:refnum<vi>)
        n346 = control-ref of="View Raw Pos."() -> (w821:refnum<vi>)
        n347 = control-ref of="Controller Gains"() -> (w822:refnum<vi>)
        n348 = case shown="True" w825 {
          tunnel: w824 -> [w843 _]
          tunnel: [w843 errorcluster {"status"=TRUE, "code"=5005, "source"="No PlaMoS file loaded!"} ("error IO")] -> w823
          frame False {
          }
          frame True {
          }
        }
        n349 = Build Array(w813, w820, w819, w818, w817, w816, w815, w814, w821, w822) -> (w812:refnum<vi>[])
        n350 = call <vilib>:"Reformat.vi"("Pretty Print Levels"=0, "error in (no error)"=w823, "JSON"=w826) -> ("error out"=w837:errorcluster, "<JSON>"=w838:string)  [unwired: 5 in, 2 out]
        n351 = for {
          tunnel: w812 -> [w847] mode=indexing
          tunnel: w823 -> [w845]
          n352 = property class="Ctl"(reference=w847, error in=w845, "DisabledEnum"=T35."Disabled and Grayed Out" ("Disabled")) -> ()  [unwired: 2 out]
        }
        n353 = call "From JSON Text.vim"("Data Type and Default Value"=T41 [] ("Planned Motion Sequence Steps"), "error in (no error)"=w837, "JSON"=w838) -> ("error out"=w829:errorcluster, "Data out"=w831:T41)  [unwired: 7 in]
        n354 = To Variant(anything=w831) -> (Variant=w832:variant)
        n355 = Bundle By Name(cluster=T32 {"Command"="", "Data"=variant} ("InterProcessQueue"), "Command"="IP: StartPlaMoS", "Data"=w832) -> (w835:T32)
        n356 = Enqueue Element(queue=w834, element=w835, error in (no error)=w829) -> (error out=w828:errorcluster)  [unwired: 1 in, 2 out]
        n357 = call <vilib>:"Add State(s) to Queue__jki_lib_state_machine.vi"("State(s) in Front (\"\")"="Config: SaveConfiguration \nStatus: Update >> Running Planned Motion Sequence" ("State(s) in Front (\"\")"), "State(s) in (\"\")"=w842) -> ("States Out"=w841:string)  [unwired: 13 in]
      }
      frame "PlaMoS: StopSequence" {
        # "Enable all controls"
        # "Load config from before\nrunning the sequence"
        # "Template Separator\n(You can make a copy of, or modify, this frame)"
        n358 = Bundle By Name(cluster=T32 {"Command"="", "Data"=variant} ("InterProcessQueue"), "Command"="IP: StopPlaMoS") -> (w865:T32)
        n359 = Enqueue Element(queue=w864, element=w865, error in (no error)=w861) -> (error out=w859:errorcluster)  [unwired: 1 in, 2 out]
        n360 = control-ref of="Reference Generation"() -> (w849:refnum<vi>)
        n361 = control-ref of="Update Controller Gains"() -> (w856:refnum<vi>)
        n362 = control-ref of="Update Reference"() -> (w855:refnum<vi>)
        n363 = control-ref of="Zero Curr. Sense"() -> (w854:refnum<vi>)
        n364 = control-ref of="Set Pos. Zero"() -> (w853:refnum<vi>)
        n365 = control-ref of="Run Controller?"() -> (w852:refnum<vi>)
        n366 = control-ref of="Set Pos. Zero"() -> (w851:refnum<vi>)
        n367 = control-ref of="Run DSA?"() -> (w850:refnum<vi>)
        n368 = control-ref of="View Raw Pos."() -> (w857:refnum<vi>)
        n369 = control-ref of="Controller Gains"() -> (w858:refnum<vi>)
        n370 = Build Array(w849, w856, w855, w854, w853, w852, w851, w850, w857, w858) -> (w848:refnum<vi>[])
        n371 = for {
          tunnel: w848 -> [w873] mode=indexing
          tunnel: w859 -> [w871]
          tunnel: [w870] -> w860
          n372 = property class="Ctl"(reference=w873, error in=w871, "DisabledEnum"=T35."Enabled" ("Disabled")) -> (error out=w870:errorcluster)  [unwired: 1 out]
        }
        n373 = call <vilib>:"Add State(s) to Queue__jki_lib_state_machine.vi"("State(s) in Front (\"\")"="Config: LoadConfiguration\n IP: UpdateCtrlGains\nStatus: Update >> Stopped Planned Motion Sequence" ("State(s) in Front (\"\")"), "State(s) in (\"\")"=w869) -> ("States Out"=w868:string)  [unwired: 13 in]
      }
      frame "---------- New Category ----------" {
        # "Template Separator\n(You can make a copy of, or modify, this frame)"
        n374 = call <vilib>:"Add State(s) to Queue__jki_lib_state_machine.vi"("State(s) in (\"\")"=w877) -> ("States Out"=w876:string)  [unwired: 14 in]
      }
      frame "New Category: 1" {
        # "Your code here.\n(You can make a copy of, or modify, this frame)"
        n375 = call <vilib>:"Add State(s) to Queue__jki_lib_state_machine.vi"("State(s) in (\"\")"=w881) -> ("States Out"=w880:string)  [unwired: 14 in]
      }
      frame "New Category: 2" {
        # "Your code here.\n(You can make a copy of, or modify, this frame)"
        n376 = call <vilib>:"Add State(s) to Queue__jki_lib_state_machine.vi"("State(s) in (\"\")"=w885) -> ("States Out"=w884:string)  [unwired: 14 in]
      }
    }
  }
  n377 = call <vilib>:"Show.vi"("error in (no error)"=w24, "SMO.UI"=w23) -> ("error out"=w54:errorcluster, "SMO.UI out"=w38:refnum<class "DisplayWaveforms.lvclass">)  [unwired: 8 in]
  n378 = while {
    tunnel: [TRUE ("Stop")] -> w32
    tunnel: w26 -> [w890]
    tunnel: w19 -> [w891]
    shift-right: [w892] -> _
    shift-left: STMLoopState_enum."Initialize" ("RTmainLoopState") -> [w893]
    shift-right: [w886] -> w16
    shift-left: w24 -> [w889]
    stop <- w887 stop-if-true
    # "Host -> Target Message Sender"
    n379 = case shown="\"Run\", Default" w893 {
      tunnel: [STMLoopState_enum."Warm-up" ("RTmainLoopState") STMLoopState_enum."Run" ("RTmainLoopState") w902 STMLoopState_enum."ShutDown" ("RTmainLoopState")] -> w892
      tunnel: w891 -> [_ _ w906 _]
      tunnel: w890 -> [_ _ w907 _]
      tunnel: w889 -> [w895 w897 w905 w1108]
      tunnel: [w895 w897 w903 w1107] -> w886
      frame "Initialize" {
      }
      frame "Warm-up" {
      }
      frame "Run", Default {
        n380 = Preview Queue Element(queue=w907, error in (no error)=w905) -> (queue out=w901:refnum<queue>, element=w899:cluster{"Command":string, "Data":variant}, error out=w904:errorcluster)  [unwired: 1 in, 1 out]
        n381 = Unbundle By Name(w899) -> ("Command"=w900:string)
        n382 = case shown="\"IP: UpdateCtrlParams\"" w900 {
          tunnel: w906 -> [_ w915 w927 w941 w955 w978 w1007 w1015 w1030 w1051 w1063 w1076 w1084 w1091 w1098 w1105]
          tunnel: w904 -> [w908 w912 w920 w936 w950 w974 w1001 w1012 w1025 w1048 w1057 w1070 w1081 w1088 w1095 w1102]
          tunnel: [w908 w914 w922 w938 w952 w976 w1003 w1014 w1027 w1050 w1059 w1072 w1083 w1090 w1097 w1104] -> w903
          tunnel: [STMLoopState_enum."Run" ("RTmainLoopState") STMLoopState_enum."Run" ("RTmainLoopState") STMLoopState_enum."Run" ("RTmainLoopState") STMLoopState_enum."Run" ("RTmainLoopState") STMLoopState_enum."Run" ("RTmainLoopState") STMLoopState_enum."Run" ("RTmainLoopState") STMLoopState_enum."Run" ("RTmainLoopState") STMLoopState_enum."Run" ("RTmainLoopState") STMLoopState_enum."Run" ("RTmainLoopState") STMLoopState_enum."Run" ("RTmainLoopState") STMLoopState_enum."Run" ("RTmainLoopState") STMLoopState_enum."Run" ("RTmainLoopState") STMLoopState_enum."Run" ("RTmainLoopState") STMLoopState_enum."Run" ("RTmainLoopState") STMLoopState_enum."Run" ("RTmainLoopState") STMLoopState_enum."ShutDown" ("RTmainLoopState")] -> w902
          tunnel: w901 -> [_ w911 w919 w935 w949 w973 w1000 w1011 w1024 w1047 w1056 w1069 w1080 w1087 w1094 w1101]
          frame "idle", Default {
          }
          frame "IP: ReadFPGActrl_loopTime" {
            n383 = Dequeue Element(queue=w911, error in (no error)=w912) -> (error out=w910:errorcluster)  [unwired: 1 in, 3 out]
            n384 = call-poly <vilib>:"Write Message.vi"("error in"=w910, "name"="PC: ReadFPGActrl_loopTime", "connection info in"=w915) -> ("error out"=w914:errorcluster)  [unwired: 7 in, 1 out]
          }
          frame "IP: SetRTtimedLoop_dt" {
            n385 = Dequeue Element(queue=w919, error in (no error)=w920) -> (element=w918:cluster{"Command":string, "Data":variant})  [unwired: 1 in, 3 out]
            n386 = Unbundle By Name(w918) -> ("Data"=w917:variant)
            n387 = Variant To Data(type=i64 0, Variant=w917) -> (data=w926:i64, error out=w924:errorcluster)  [unwired: 1 in]
            n388 = Flatten To String(anything=w926, error in (no error)=w924) -> (data string=w929:string, error out=w923:errorcluster)  [unwired: 2 in, 1 out]
            n389 = call-poly <vilib>:"Write Message.vi"("error in"=w923, "data"=w929, "name"="PC: Set RTmain_loopTime", "connection info in"=w927) -> ("error out"=w922:errorcluster)  [unwired: 6 in, 1 out]
          }
          frame "IP: UpdateCtrlParams" {
            n390 = Dequeue Element(queue=w935, error in (no error)=w936) -> (element=w934:cluster{"Command":string, "Data":variant}, error out=w930:errorcluster)  [unwired: 1 in, 2 out]
            n391 = Unbundle By Name(w934) -> ("Data"=w933:variant)
            n392 = Variant To Data(error in=w930, type=T2 {"Z-direction"={"Kp"=1.0, "Ki"=50.0, "fLPF"=0.0}, "ThX-direction"={"Kp"=1.0, "Ki"=0.0, "fLPF"=0.0}, "ThY-direction"={"Kp"=1.0, "Ki"=0.0, "fLPF"=0.0}, "Bow-direction"={"Kp"=1.0, "Ki"=0.0, "fLPF"=0.0}, "B-d - direction"={"Kp"=0.0, "Ki"=0.0, "fLPF"=0.0}} ("Controller Gains"), Variant=w933) -> (data=w931:T2, error out=w940:errorcluster)
            n393 = Flatten To String(anything=w931, error in (no error)=w940) -> (data string=w943:string, error out=w939:errorcluster)  [unwired: 2 in, 1 out]
            n394 = call-poly <vilib>:"Write Message.vi"("error in"=w939, "data"=w943, "name"="PC: UpdateCtrlParams", "connection info in"=w941) -> ("error out"=w938:errorcluster)  [unwired: 6 in, 1 out]
          }
          frame "IP: SetFPGAPosZeroOffset" {
            n395 = Dequeue Element(queue=w949, error in (no error)=w950) -> (element=w948:cluster{"Command":string, "Data":variant}, error out=w944:errorcluster)  [unwired: 1 in, 2 out]
            n396 = Unbundle By Name(w948) -> ("Data"=w947:variant)
            n397 = Variant To Data(error in=w944, type=T20 {"V_SE"=0.0, "V_NE"=0.0, "V_NW"=0.0, "V_SW"=0.0, "V_CI"=0.0} ("Pos Zero Offsets [V]"), Variant=w947) -> (data=w946:T20, error out=w954:errorcluster)
            n398 = Flatten To String(anything=w946, error in (no error)=w954) -> (data string=w957:string, error out=w953:errorcluster)  [unwired: 2 in, 1 out]
            n399 = call-poly <vilib>:"Write Message.vi"("error in"=w953, "data"=w957, "name"="PC: SetFPGAPosZeroOffset", "connection info in"=w955) -> ("error out"=w952:errorcluster)  [unwired: 6 in, 1 out]
          }
          frame "IP: UpdateReference" {
            # "Scale Amplitude to set based on\nZ, Th multipliers"
            n400 = local read "Coord. Trans. Multipliers"() -> (w965:T13)
            n401 = Dequeue Element(queue=w973, error in (no error)=w974) -> (element=w972:cluster{"Command":string, "Data":variant}, error out=w967:errorcluster)  [unwired: 1 in, 2 out]
            n402 = Unbundle By Name(w972) -> ("Data"=w971:variant)
            n403 = Variant To Data(error in=w967, type=T33 {"Reference Location"=enum."Pos Ref", "Direction"=enum."Z", "Excitation mode"=enum."DC", "Amplitude"=0.0, "Frequency (periods/tick)"=0.0, "PosRef_Offset"=[]} ("FuncGen Params"), Variant=w971) -> (data=w968:T33)  [unwired: 1 out]
            n404 = Unbundle By Name(w968) -> ("Reference Location"=w969:T5, "Direction"=w966:T10, "PosRef_Offset"=w964:dbl[])
            n405 = Unbundle By Name(w965) -> ("Z"=w958:dbl, "Th"=w962:dbl)
            n406 = Build Array(w958, w962, w962, w958, w958) -> (w963:dbl[])
            n407 = case shown="\"Pos Ref\"" w969 {
              tunnel: w968 -> [w984 w996]
              tunnel: [w982 w996] -> w961
              tunnel: w966 -> [w985 _]
              tunnel: w958 -> [w983 _]
              tunnel: w962 -> [w981 _]
              frame "Pos Ref" {
                n408 = case shown="\"Z\", \"Bow\", Default" w985 {
                  tunnel: w984 -> [w988 w995]
                  tunnel: w983 -> [w989 _]
                  tunnel: [w986 w994] -> w982
                  tunnel: w981 -> [_ w991]
                  frame "Z", "Bow", Default {
                    n409 = Unbundle By Name(w988) -> ("Amplitude"=w990:dbl)
                    n410 = Divide(x=w990, y=w989) -> (x/y=w987:dbl)
                    n411 = Bundle By Name(cluster=w988, "Amplitude"=w987) -> (w986:T33)
                  }
                  frame "ThX", "ThY" {
                    n412 = Unbundle By Name(w995) -> ("Amplitude"=w993:dbl)
                    n413 = Divide(x=w993, y=w991) -> (x/y=w992:dbl)
                    n414 = Bundle By Name(cluster=w995, "Amplitude"=w992) -> (w994:T33)
                  }
                }
              }
              frame "Ctrl Eff", Default {
              }
            }
            n415 = Divide(x=w964, y=w963) -> (x/y=w960:dbl[])
            n416 = Bundle By Name(cluster=w961, "PosRef_Offset"=w960) -> (w959:T33)
            n417 = Flatten To String(anything=w959) -> (data string=w980:string, error out=w977:errorcluster)  [unwired: 3 in, 1 out]
            n418 = call-poly <vilib>:"Write Message.vi"("error in"=w977, "data"=w980, "name"="PC: UpdateReference", "connection info in"=w978) -> ("error out"=w976:errorcluster)  [unwired: 6 in, 1 out]
          }
          frame "IP: StartDSA" {
            n419 = Dequeue Element(queue=w1000, error in (no error)=w1001) -> (element=w999:cluster{"Command":string, "Data":variant})  [unwired: 1 in, 3 out]
            n420 = Unbundle By Name(w999) -> ("Data"=w998:variant)
            n421 = Variant To Data(type=T36 {"DSA excitation specs"={"Initial Freq. [Hz]"=1.0, "Final Freq. [Hz]"=100.0, "# pts. in interval"=20, "Samping Time [us]"=0.0, "Amplitude"=0.0003, "Offset [V]"=0.0, "Freq Units (F: rad/s, T: Hz)"=TRUE}, "Cycle Specs"={"Cycles To \nSettle (M)"=1, "Cycles To \nCalculate (N)"=2}, "Meas. TF params"={"Direction"=enum."Z", "Tras. Func."=enum."P"}} ("DSA Config Cluster"), Variant=w998) -> (data=w1006:T36, error out=w1005:errorcluster)  [unwired: 1 in]
            n422 = Flatten To String(anything=w1006, error in (no error)=w1005) -> (data string=w1009:string, error out=w1004:errorcluster)  [unwired: 2 in, 1 out]
            n423 = call-poly <vilib>:"Write Message.vi"("error in"=w1004, "data"=w1009, "name"="PC: StartDSA", "connection info in"=w1007) -> ("error out"=w1003:errorcluster)  [unwired: 6 in, 1 out]
          }
          frame "IP: StopDSA" {
            n424 = Dequeue Element(queue=w1011, error in (no error)=w1012) -> (error out=w1010:errorcluster)  [unwired: 1 in, 3 out]
            n425 = call-poly <vilib>:"Write Message.vi"("error in"=w1010, "name"="PC: StopDSA", "connection info in"=w1015) -> ("error out"=w1014:errorcluster)  [unwired: 7 in, 1 out]
          }
          frame "IP: StartPlaMoS" {
            # "#TODO: Scale Amplitude to set based on\nZ, Bow before sending to RT target!"
            n426 = local read "Coord. Trans. Multipliers"() -> (w1019:T13)
            n427 = Dequeue Element(queue=w1024, error in (no error)=w1025) -> (element=w1023:cluster{"Command":string, "Data":variant})  [unwired: 1 in, 3 out]
            n428 = Unbundle By Name(w1023) -> ("Data"=w1022:variant)
            n429 = Variant To Data(type=T41 [] ("Planned Motion Sequence Steps"), Variant=w1022) -> (data=w1020:T41, error out=w1029:errorcluster)  [unwired: 1 in]
            n430 = Unbundle By Name(w1019) -> ("Z"=w1018:dbl)
            n431 = for {
              tunnel: w1020 -> [w1045] mode=indexing
              tunnel: w1018 -> [w1041]
              tunnel: [w1035] -> w1017 mode=indexing
              n432 = Unbundle By Name(w1045) -> ("StepParams.PosCtrl Params.Velocity [um/s]"=w1034:dbl, "StepParams.PosCtrl Params.Starting Z-position [um]"=w1044:dbl, "StepParams.PosCtrl Params.Ending Z-position [um]"=w1043:dbl, "StepParams.PosCtrl Params.Bow Reference [um]"=w1042:dbl)
              n433 = Build Array(w1034, w1044, w1043, w1042) -> (w1040:dbl[])
              n434 = Divide(x=w1040, y=w1041) -> (x/y=w1039:dbl[])
              n435 = Index Array(array=w1039) -> (element #1=w1038:dbl, element #2=w1037:dbl, element #3=w1036:dbl, element #4=w1033:dbl)  [unwired: 4 in]
              n436 = Bundle By Name(cluster=w1045, "StepParams.PosCtrl Params.Velocity [um/s]"=w1038, "StepParams.PosCtrl Params.Starting Z-position [um]"=w1037, "StepParams.PosCtrl Params.Ending Z-position [um]"=w1036, "StepParams.PosCtrl Params.Bow Reference [um]"=w1033) -> (w1035:T42)
            }
            n437 = Flatten To String(anything=w1017, error in (no error)=w1029) -> (data string=w1032:string, error out=w1028:errorcluster)  [unwired: 2 in, 1 out]
            n438 = call-poly <vilib>:"Write Message.vi"("error in"=w1028, "data"=w1032, "name"="PC: StartPlaMoS", "connection info in"=w1030) -> ("error out"=w1027:errorcluster)  [unwired: 6 in, 1 out]
          }
          frame "IP: StopPlaMoS" {
            n439 = Dequeue Element(queue=w1047, error in (no error)=w1048) -> (error out=w1046:errorcluster)  [unwired: 1 in, 3 out]
            n440 = call-poly <vilib>:"Write Message.vi"("error in"=w1046, "name"="PC: StopPlaMoS", "connection info in"=w1051) -> ("error out"=w1050:errorcluster)  [unwired: 7 in, 1 out]
          }
          frame "IP: AOenable" {
            n441 = Dequeue Element(queue=w1056, error in (no error)=w1057) -> (element=w1055:cluster{"Command":string, "Data":variant})  [unwired: 1 in, 3 out]
            n442 = Unbundle By Name(w1055) -> ("Data"=w1054:variant)
            n443 = Variant To Data(type=FALSE, Variant=w1054) -> (data=w1062:bool, error out=w1061:errorcluster)  [unwired: 1 in]
            n444 = Flatten To String(anything=w1062, error in (no error)=w1061) -> (data string=w1065:string, error out=w1060:errorcluster)  [unwired: 2 in, 1 out]
            n445 = call-poly <vilib>:"Write Message.vi"("error in"=w1060, "data"=w1065, "name"="PC: AOenable", "connection info in"=w1063) -> ("error out"=w1059:errorcluster)  [unwired: 6 in, 1 out]
          }
          frame "IP: RunCtrl" {
            n446 = Dequeue Element(queue=w1069, error in (no error)=w1070) -> (element=w1068:cluster{"Command":string, "Data":variant})  [unwired: 1 in, 3 out]
            n447 = Unbundle By Name(w1068) -> ("Data"=w1067:variant)
            n448 = Variant To Data(type=FALSE, Variant=w1067) -> (data=w1075:bool, error out=w1074:errorcluster)  [unwired: 1 in]
            n449 = Flatten To String(anything=w1075, error in (no error)=w1074) -> (data string=w1078:string, error out=w1073:errorcluster)  [unwired: 2 in, 1 out]
            n450 = call-poly <vilib>:"Write Message.vi"("error in"=w1073, "data"=w1078, "name"="PC: RunCtrl", "connection info in"=w1076) -> ("error out"=w1072:errorcluster)  [unwired: 6 in, 1 out]
          }
          frame "IP: ResetZeroPosition" {
            n451 = Dequeue Element(queue=w1080, error in (no error)=w1081) -> (error out=w1079:errorcluster)  [unwired: 1 in, 3 out]
            n452 = call-poly <vilib>:"Write Message.vi"("error in"=w1079, "name"="PC: ResetZeroPosition", "connection info in"=w1084) -> ("error out"=w1083:errorcluster)  [unwired: 7 in, 1 out]
          }
          frame "IP: ViewRawPosition" {
            n453 = Dequeue Element(queue=w1087, error in (no error)=w1088) -> (error out=w1086:errorcluster)  [unwired: 1 in, 3 out]
            n454 = call-poly <vilib>:"Write Message.vi"("error in"=w1086, "name"="PC: ViewRawPosition", "connection info in"=w1091) -> ("error out"=w1090:errorcluster)  [unwired: 7 in, 1 out]
          }
          frame "IP: ResetZeroCurrSense" {
            n455 = Dequeue Element(queue=w1094, error in (no error)=w1095) -> (error out=w1093:errorcluster)  [unwired: 1 in, 3 out]
            n456 = call-poly <vilib>:"Write Message.vi"("error in"=w1093, "name"="PC: ResetZeroCurrSense", "connection info in"=w1098) -> ("error out"=w1097:errorcluster)  [unwired: 7 in, 1 out]
          }
          frame "IP: ShutDown" {
            n457 = Dequeue Element(queue=w1101, error in (no error)=w1102) -> (error out=w1100:errorcluster)  [unwired: 1 in, 3 out]
            n458 = call-poly <vilib>:"Write Message.vi"("error in"=w1100, "name"="PC: ShutDown", "connection info in"=w1105) -> ("error out"=w1104:errorcluster)  [unwired: 7 in, 1 out]
          }
        }
      }
      frame "ShutDown" {
        n459 = shared-variable ".\\Variables.lvlib\\Stop"(TRUE ("Stop"), error in=w1108) -> (error out=w1107:errorcluster)
      }
    }
    n460 = shared-variable ".\\Variables.lvlib\\Stop"() -> (w888:bool)  [unwired: 1 in, 1 out]
    n461 = Or(x=w886, y=w888) -> (x .or. y?=w887:bool)
  }
  n462 = while {
    tunnel: [TRUE ("Stop")] -> w31
    tunnel: w19 -> [w1117]
    shift-right: [w1116] -> _
    shift-left: STMLoopState_enum."Initialize" ("RTmainLoopState") -> [w1118]
    shift-right: [w1112] -> w17
    shift-left: w24 -> [w1115]
    tunnel: w5 -> [w1111]
    stop <- w1113 stop-if-true
    # "Target -> Host Message Parser"
    n463 = case shown="\"Run\", Default" w1118 {
      tunnel: w1117 -> [_ _ w1131 _]
      tunnel: [STMLoopState_enum."Warm-up" ("RTmainLoopState") STMLoopState_enum."Run" ("RTmainLoopState") STMLoopState_enum."Run" ("RTmainLoopState") STMLoopState_enum."ShutDown" ("RTmainLoopState")] -> w1116
      tunnel: w1115 -> [w1120 w1122 w1130 w1185]
      tunnel: [w1120 w1122 w1125 w1185] -> w1112
      tunnel: w1111 -> [_ _ w1124 _]
      frame "Initialize" {
      }
      frame "Warm-up" {
      }
      frame "Run", Default {
        n464 = call-poly <vilib>:"Read Message.vi"("options"=T52 {"ignore timeout error"=TRUE, "timeout ms (1000)"=1000}, "error in"=w1130, "connection info in"=w1131) -> ("error out"=w1128:errorcluster, "name"=w1127:T27, "data string"=w1126:string, "timed out?"=w1129:bool)  [unwired: 2 in, 3 out]
        n465 = case shown="False" w1129 {
          tunnel: w1128 -> [w1136 w1184]
          tunnel: w1127 -> [w1138 _]
          tunnel: w1126 -> [w1137 _]
          tunnel: [w1135 w1184] -> w1125
          tunnel: w1124 -> [w1134 _]
          frame False {
            n466 = case shown="\"RT: GetBodeData\"" w1138 {
              tunnel: w1137 -> [_ w1143 w1149 w1154 w1168 _ w1179 w1182]
              tunnel: w1136 -> [w1139 w1141 w1148 w1153 w1167 w1169 w1178 w1183]
              tunnel: [w1139 w1140 w1147 w1152 w1155 w1170 w1175 w1183] -> w1135
              tunnel: w1134 -> [_ _ _ _ _ _ w1174 _]
              frame "idle", Default {
              }
              frame "RT: GetFPGActrl_loopTime" {
                n467 = Unflatten From String(type=0.0, binary string=w1143, error in (no error)=w1141) -> (value=w1142:dbl, error out=w1140:errorcluster)  [unwired: 2 in, 1 out]
                n468 = local write "FPGA Controller Loop Time [us]"(w1142) -> ()
              }
              frame "RT: GetZeroPosOffsets" {
                n469 = Unflatten From String(type=T53 {"V_SE"=0.0, "V_NE"=0.0, "V_NW"=0.0, "V_SW"=0.0, "V_CI"=0.0} ("Zero Offsets [V]"), binary string=w1149, error in (no error)=w1148) -> (value=w1145:T53, error out=w1147:errorcluster)  [unwired: 2 in, 1 out]
                n470 = local write "Pos Zero Offsets [V]"(w1145) -> ()
              }
              frame "RT: GetZeroCurrSense" {
                n471 = Unflatten From String(type=T54 {"I_SE"=0.0, "I_NE"=0.0, "I_NW"=0.0, "I_SW"=0.0, "I_CO"=0.0, "I_CI"=0.0} ("Curr Sense Zero [mA]"), binary string=w1154, error in (no error)=w1153) -> (value=w1151:T54, error out=w1152:errorcluster)  [unwired: 2 in, 1 out]
                n472 = local write "Curr Sense Zero [mA]"(w1151) -> ()
              }
              frame "RT: GetBodeData" {
                # "Reset Control State and \nenable DSA excitation cluster"
                n473 = Unflatten From String(type=T40 {"Frequency [Hz]"=[], "Magnitude [abs]"=[], "Phase [deg]"=[]} ("Bode Plots"), binary string=w1168, error in (no error)=w1167) -> (value=w1165:T40, error out=w1161:errorcluster)  [unwired: 2 in, 1 out]
                n474 = Unbundle(w1165) -> ("Frequency [Hz]"=w1164:dbl[], "Magnitude [abs]"=w1163:dbl[], "Phase [deg]"=w1160:dbl[])
                n475 = property on="Run DSA?" class="Bool (strict)"(error in=w1161, "Val(Sgnl)"=FALSE ("Value (Signaling)")) -> (error out=w1155:errorcluster)  [unwired: 1 in, 1 out]
                n476 = Bundle("Frequency [Hz]"=w1164, "Magnitude [abs]"=w1163) -> (w1158:T55)  [unwired: 1 in]
                n477 = Bundle("Frequency [Hz]"=w1164, "Phase [deg]"=w1160) -> (w1157:T56)  [unwired: 1 in]
                n478 = Bundle(cluster=T8 {"Magnitude Bode Plot"={[1.0, 1.2742749857031337, 1.6237767391887217, 2.0691380811147897, 2.636650898730358, 3.3598182862837818, 4.281332398719393, 5.455594781168519, 6.951927961775605, 8.858667904100825, 11.28837891684689, 14.38449888287663, 18.329807108324356, 23.357214690901213, 29.76351441631318, 37.926901907322495, 48.32930238571752, 61.584821106602604, 78.47599703514611, 100.0], [8.190036284839644, 6.422876871403994, 5.062364967545408, 4.022651018777153, 3.220267625701321, 2.6042578837321395, 2.1431756051838486, 1.7956979443459349, 1.5432350752401756, 1.3654027683935595, 1.2417506496398736, 1.1608055133183222, 1.1086862764056675, 1.0725909164599179, 1.0432556265245092, 1.0364066986654934, 1.0216396632894174, 1.0177430021270428, 1.0137984534990414, 1.0067815519527075]}, "Phase Bode Plot"={[1.0, 1.2742749857031337, 1.6237767391887217, 2.0691380811147897, 2.636650898730358, 3.3598182862837818, 4.281332398719393, 5.455594781168519, 6.951927961775605, 8.858667904100825, 11.28837891684689, 14.38449888287663, 18.329807108324356, 23.357214690901213, 29.76351441631318, 37.926901907322495, 48.32930238571752, 61.584821106602604, 78.47599703514611, 100.0], [-81.48463378500874, -79.51768777854348, -77.26541119865844, -74.35073441612305, -70.71358924826187, -66.32524067891468, -60.91360319984072, -54.8342286888728, -48.311197626693605, -41.59636553315517, -34.99300908851906, -29.13860750441638, -24.098834956322154, -19.566458637535703, -14.982365658719985, -13.159615969942717, -9.781179665619796, -8.18372823642157, -6.386288856595014, -4.541305979436174]}} ("Bode Data"), "Magnitude Bode Plot"=w1158, "Phase Bode Plot"=w1157) -> (→"Bode Data":T8)
              }
              frame "RT: StoppedPlaMoS" {
                # "Go back to how UI \nwas before sequence\n\nLast controller state in FPGA is maintained,\nOnly UI is updated."
                n479 = property on="Run Plannned Motion Sequence?" class="Bool (strict)"(error in=w1169, "Val(Sgnl)"=FALSE ("Value (Signaling)")) -> (error out=w1170:errorcluster)  [unwired: 1 in, 1 out]
              }
              frame "RT: UpdateDispWaveform" {
                # "Scale Z, Th scales with multiplier before plotting \nin the Chart Process VI - see chart process VI"
                # "#TODO: How to pass display data by reference\nto the display process VI?"
                n480 = Unflatten From String(type=dbl[][] [], binary string=w1179, error in (no error)=w1178) -> (value=w1172:dbl[][], error out=w1177:errorcluster)  [unwired: 2 in, 1 out]
                n481 = Array Size(array=w1172) -> (size(s)=→"# of display elements \nunpacked (row x col)":i32[])
                n482 = Generate User Event(user event=w1174, event data cluster=w1172, error in=w1177) -> (error out=w1175:errorcluster)  [unwired: 1 in, 1 out]
              }
              frame "RT: Error" {
                n483 = Concatenate Strings("RT Error: " ("string"), w1182) -> (w1180:string)
                n484 = local write "Status"(w1180) -> ()
              }
            }
          }
          frame True {
          }
        }
      }
      frame "ShutDown" {
      }
    }
    n485 = shared-variable ".\\Variables.lvlib\\Stop"() -> (w1114:bool)  [unwired: 1 in, 1 out]
    n486 = Or(x=w1112, y=w1114) -> (x .or. y?=w1113:bool)
  }
  n487 = shared-variable ".\\Variables.lvlib\\Stop"(w33) -> ()  [unwired: 1 in, 1 out]
  n488 = Unregister For Events(event registration refnum=w35) -> (error out=w57:errorcluster)  [unwired: 1 in]
  n489 = Merge Errors(w4, w54) -> (w34:errorcluster)
  n490 = shared-variable ".\\Variables.lvlib\\Stop"(w31) -> ()  [unwired: 1 in, 1 out]
  n491 = Merge Errors(w17, w16) -> (w18:errorcluster)
  n492 = shared-variable ".\\Variables.lvlib\\Stop"(w32) -> ()  [unwired: 1 in, 1 out]
  n493 = call <vilib>:"Destroy.vi"("error in (no error)"=w34, "SMO"=w38) -> ("error out"=w56:errorcluster)  [unwired: 9 in]
  n494 = call-poly <vilib>:"Get Connection Reference.vi"("error in"=w18, "connection info in"=w19) -> ("error out"=w22:errorcluster, "connection ID out"=w20:refnum<k5>)  [unwired: 7 in, 1 out]
  n495 = TCP Close Connection(connection ID=w20, error in (no error)=w22) -> (error out=w21:errorcluster)  [unwired: 1 in, 1 out]
  n496 = call "Specific Error Handler"("Error to Check"=w21) -> ("error out"=w3:errorcluster)  [unwired: 11 in, 3 out]
  n497 = property on="Stop" class="Bool (strict)"(error in=w3, "Val(Sgnl)"=TRUE ("Value (Signaling)")) -> (error out=w2:errorcluster)  [unwired: 1 in, 1 out]
  n498 = Merge Errors(w57, w56, w2) -> (w15:errorcluster)
  n499 = call "Close Queues.vi"("error in (no error)"=w15, "FIFOs In"=w9) -> ("error out"=w14:errorcluster)  [unwired: 9 in]
  n500 = call <vilib>:"Simple Error Handler.vi"("error in (no error)"=w14) -> ()  [unwired: 4 in, 5 out]
